vi "Tracker.vi"() -> ()   [LabVIEW 2016]
uses:
  Globaltracker.vi
panel:
  in  "EXPORT 2":enum16{"RAW", "TXT", "CSV"}(ring)
  out "TotalDistanceTraveled":dbl=0.1124215336624257
  out "SegmentsRecalculation":bool[](array[boolean])
  out "ForAnalysisLastRecordingPath":path=path "D:/Users/Dmitriy/CData/CloudStation/Tracker_repository/SavedTrack-2018-02-26-17-00-54/SavedTrack-2018-02-26-17-00-54.csv"
  in  "i":i32=113
  out "NotificationCount":i32
  out "Alarm":dbl caption="minutes" format="%#g"
  out "Loadedregions":picture
  out "Mousebackground":picture
  out "OutsideaSegment":dbl[](array[slide]) scale=-1.0..83.73750000001033
  out "InsideaSegment":dbl[](array[slide]) scale=-1.0..83.73750000001033
  out "TtlArray":T1(array[cluster])
  in  "Main TabControl":enum32{"Settings", "Recording", "Analysis"}(tab)
  in  "CageSegmentation":enum32{"Page 1", "Page 2"}(tab)
  in  "Startup via TTL input 2":bool
  in  "Start/stop signaling":bool=TRUE
  out "CageSegmentation":string="Cage Segmentation"
  out "AssignedSegments":string="Assigned Segments:"
  in  "ListboxOfSegments":i32(listbox)
  in  "Border":enum32{"Page 1", "Page 2"}(tab)
  out "Border":string="BORDER"
  in  "Border":enum16{"8", "6", "5", "4", "3", "2", "1", "0"}(ring)=enum."4" caption="Number of\n segments"
  in  "StartingAngleBorder":u16 caption="Starting\n angle" max=360 step=1
  in  "Center":enum32{"Page 1", "Page 2"}(tab)
  in  "Center":enum16{"1", "0"}(ring) caption="Number of\n segments"
  in  "RadiusCenter":u16=25 caption="Radius \n (mm)" max=90
  out "Center":string="CENTER"
  in  "Midfield":enum32{"Page 1", "Page 2"}(tab)
  in  "StartingAngleMidfield":u32 caption="Starting\n angle" max=360 step=1
  in  "RadiusMidfield":u16=55 caption="Radius\n (mm)" max=90 step=1
  in  "Midfield":enum16{"4", "3", "2", "1", "0"}(ring)=enum."1" caption="Number of\n segments"
  out "Midfiled":string="MIDFIELD"
  out "SettingsDisplay":picture
  out "?":picture
  in  "KeyboardShortcuts":enum32{"Page 1", "Page 2"}(tab)
  out "KeyboardShortcuts":string="Keyboard Shortcuts"
  out "_Assigning Buttons_":bool
  in  "KeyBoardShortCuts":bool
  in  "Notifications":enum32{"Page 1", "Page 2"}(tab)
  out "Notifications":string="Notifications"
  out "Notification":bool
  in  "NotificationsON":bool
  in  "FilterType":enum32{"Page 1", "Page 2"}(tab)
  out "FIlterType":string="Filter Type"
  in  "FilterType":enum16{"No filter", "Kalman filter"}(ring)=enum."Kalman filter"
  in  "PortSelection":enum32{"Page 1", "Page 2"}(tab)
  out "PortSelection":string="Port Selection"
  in  "Data Port Selection":refnum<visa-resource-name>="Tracker"
  in  "SAVE":bool=TRUE
  out "?":picture
  in  "KeyboardShortcuts":enum32{"Page 1", "Page 2"}(tab)
  in  "SegmentsMulticolumnListbox":i32(listbox)
  out "KeyboardShortcuts":string="Keyboard Shortcuts"
  out "Notification":bool
  out "RecordingDisplay":picture
  in  "Cage Segments":enum32{"Page 1", "Page 2"}(tab)
  out "Segments(s)":dbl[](array[slide])=[0.0, 0.0, 0.0, 0.0, 0.0, 4.212500000000026] scale=-1.0..16.81249999999958
  out "Segments":bool[](array[boolean])=[FALSE, FALSE, FALSE, FALSE, FALSE, TRUE]
  out "1":string="1"
  out "2":string="2"
  out "3":string="3"
  out "4":string="4"
  out "5":string="5"
  out "6":string="6"
  out "7":string="7"
  out "8":string="8"
  out "9":string="9"
  out "10\n10":string="10"
  out "11":string="11"
  out "12":string="12"
  out "13":string="13"
  out "CageSegments":string="Cage Segments"
  in  "Cage orientation swap":bool caption="Swap coords"
  in  "RecordingTab":enum32{"Page 1", "Page 2"}(tab)
  out "TTL1 rec armed":bool=TRUE
  in  "Stop Button":bool
  in  "Start":bool
  in  "Trace length (s)":dbl(slide) scale=0.0..10.0
  in  "DisplaySegments":enum32{"Page 1", "Page 2"}(tab)
  in  "DisplaySegments":bool caption="Display Segments"
  out "DisplaySegments":string="Display \nSegments"
  in  "CurrentDistanceTraveled":enum32{"Page 1", "Page 2"}(tab)
  out "Current distance\n traveled (m)":dbl(slide)=0.1124215336624257 scale=0.0..8.0
  out "CurrentDistanceTraveled":string="Current Distance Traveled"
  in  "ElapsedTimeRecording":enum32{"Page 1", "Page 2"}(tab)
  out "Time1":string="           HH:MM:SS,MS"
  out "Time elapsed":string="00:00:04,754"
  out "ElapsedTimeRecording":string="  Elapsed Time (recording)"
  out "Mouse speed (cm/s)":dbl(knob)=3.912345932114511 scale=0.0..100.0 scale format="%#_6f"
  out "Mouse speed (cm/s)  2":dbl(graph)=3.912345932114511 caption="Mouse speed plotted vs time"
  in  "LoadRecording":enum32{"Page 1", "Page 2"}(tab)
  out "FileName":string
  out "ProgressBar":u16(slide) scale=0.0..100.0
  in  "LOAD RECORDING":bool
  in  "ElapsedTimePlayback":enum32{"Page 1", "Page 2"}(tab)
  out "Time2":string="           HH:MM:SS,MS"
  out "ElapsedTimePlayback":string="  Elapsed Time (playback)"
  out "date/time":string
  in  "PlaybackControl":enum32{"Page 1", "Page 2"}(tab)
  in  "Stop Button":bool
  in  "Start/play":bool
  in  "Skip Back Button":bool
  in  "Seek Back Button":bool
  in  "Seek Forward Button":bool
  in  "Skip Forward Button":bool
  in  "Playback progress (min)":dbl(slide) min=0.0 max=24.0 scale=0.0..1.0
  out "Display Speed":dbl
  out "Playback Speed":string="1 X"
  in  "SubtractButton":bool
  in  "AddButton":bool
  out "AnalysisDisplay":picture
  out "Mouse Speed plotted vs time":dbl(graph) caption="Mouse Speed Plotted vs Time"
  out "Mouse speed (cm/s)":dbl(knob) scale=0.0..100.0
  in  "DisplayOptions":enum32{"Page 1", "Page 2"}(tab)
  in  "Heat Map":bool
  in  "Trace_length (s)":dbl(slide) scale=0.0..10.0
  in  "FullTrack":bool caption="Full Track"
  in  "SegmentsOn":bool caption="Segments"
  out "DisplayOptions":string="Display Options"
  in  "Statistics":enum32{"Page 1", "Page 2"}(tab)
  out "Current Distance\n Traveled (m)":dbl(slide) scale=0.0..2.0 scale format="%#_6f"
  out "Total Distance Traveled (m)":dbl
  out "Average Speed (cm/s)":dbl
  out "TTL":bool
  out "Statitics":string="Statistics"
  in  "EXIT":bool=TRUE
  out "index":i32
  out "?":picture
  in  "TimeSpentinEachSegment":enum32{"Page 1", "Page 2"}(tab)
  out "TimeSpentinEachSegment":string="Time Spent in Each Segment"
  in  "TimeSpentinEachSegmentMultiListBox":i32(listbox)=-1
  out "Heat-Map":dbl[][](graph)
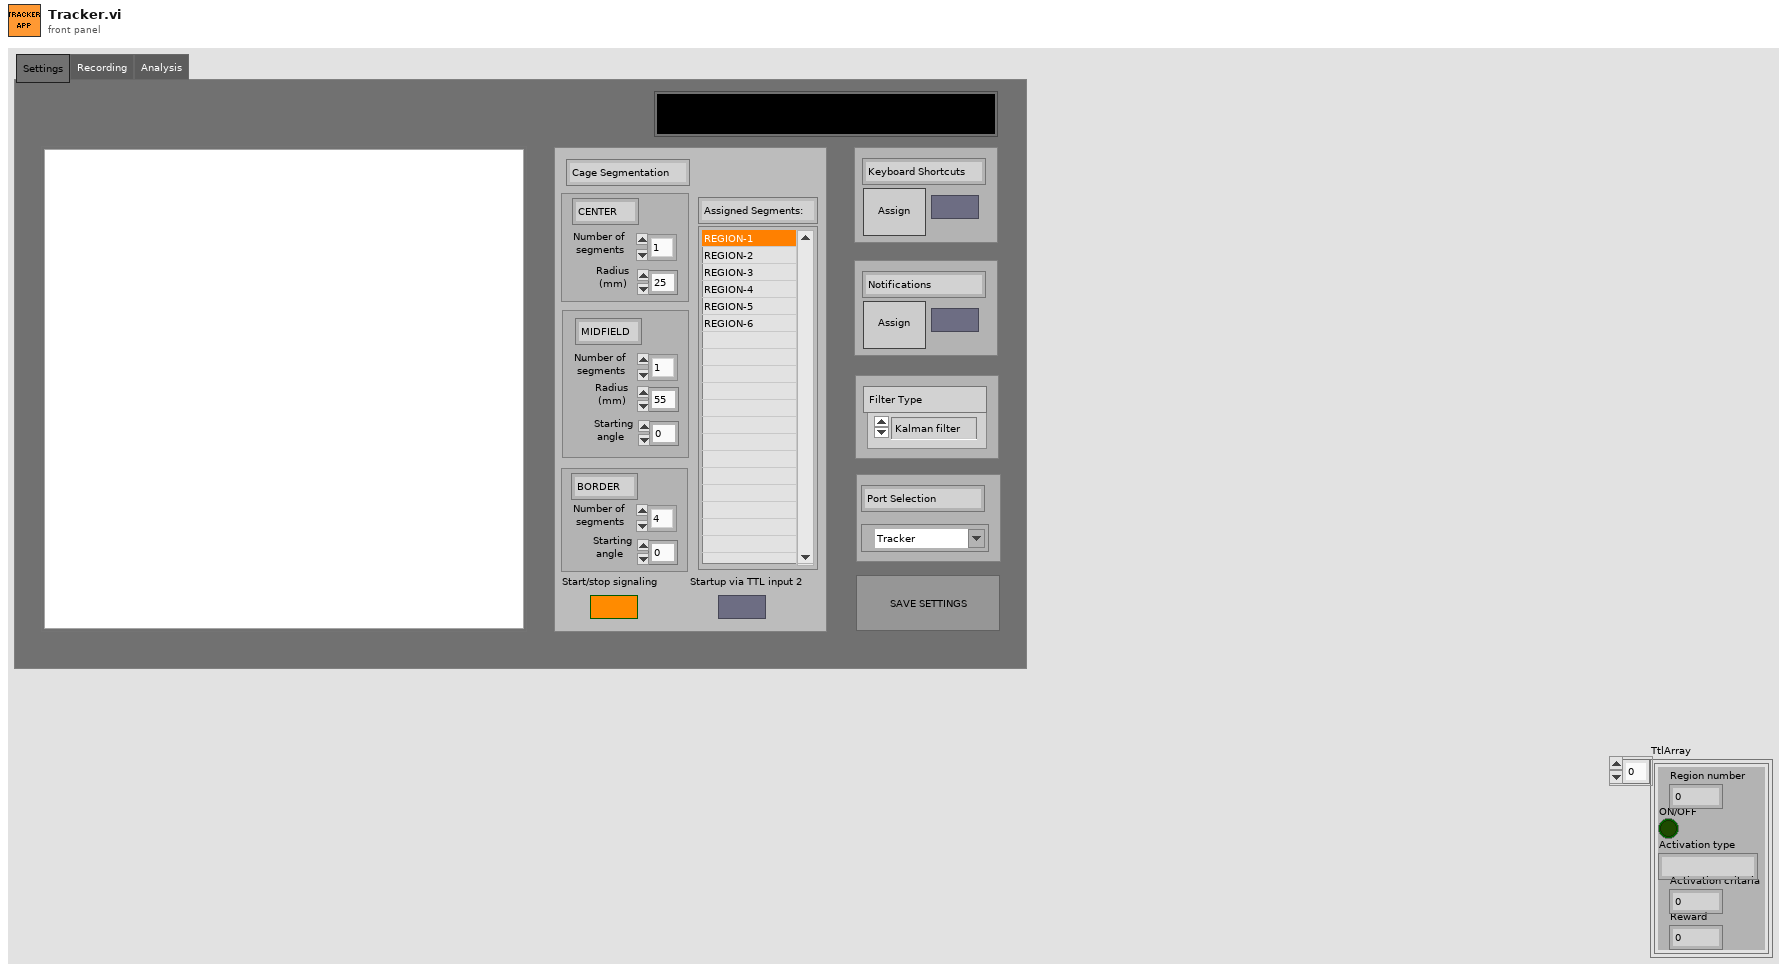
[diagram p1: front panel]
types:
  T1 = cluster{"Region number":i32, "ON/OFF":bool, "Activation type":string, "Activation critaria":i32, "Reward":i32}[]
  T2 = enum16{"No filter", "Kalman filter", "Thresholding"}
  T3 = enum8{"Enabled", "Disabled", "Disabled and Grayed Out"}
  T4 = cluster{"Starting degree of walll":u16, "RewardSystem-ON/OFF":bool, "Image Name":string, "Starting degree of walll":u16, "Starting degree of walll":u16}
  T5 = cluster{"Starting degree of walll":u16, "RewardSystem-ON/OFF":bool, "Image Name":string, "Starting degree of walll":u16, "Starting degree of walll":u16}[]
  T6 = cluster{i32, "ON-OFF":bool, "Activation":string, "ActivationCritaria":i32, "TTLActivation":i32}
  T7 = typedef "imagedata.ctl" = cluster{"image type":i32, "image depth":i32, "image":u8[], "mask":u8[], "colors":u32[], "Rectangle":cluster{"left":i16, "top":i16, "right":i16, "bottom":i16}}
  T8 = typedef "LVMouseTypeDef.ctl" = cluster{"Mouse Position":cluster{"X":i32, "Y":i32}, "Mouse Modifiers":cluster{"Button Down":bool, "Shift Mod":bool, "Menu Mod":bool, "Option Mod":bool}}
  T9 = enum32{"invalid app kind", "Development System", "Run Time System", "Student Edition", "Embedded LabVIEW", "Evaluation", "Custom"}
  T10 = typedef "LVDateTimeRec.ctl" = cluster{"fractional second":dbl, "second":i32, "minute":i32, "hour":i32, "day of month":i32, "month":i32, "year":i32, "day of week":i32, "day of year":i32, "DST":i32}
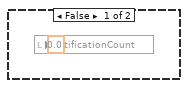
[diagram p2: hidden frame]
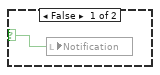
[diagram p4: hidden frame]
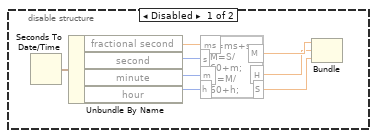
[diagram p6: hidden frame]
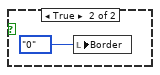
[diagram p9: hidden frame]
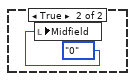
[diagram p10: hidden frame]
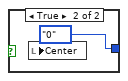
[diagram p11: hidden frame]
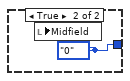
[diagram p12: hidden frame]
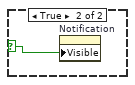
[diagram p14: hidden frame]
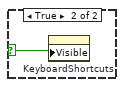
[diagram p15: hidden frame]
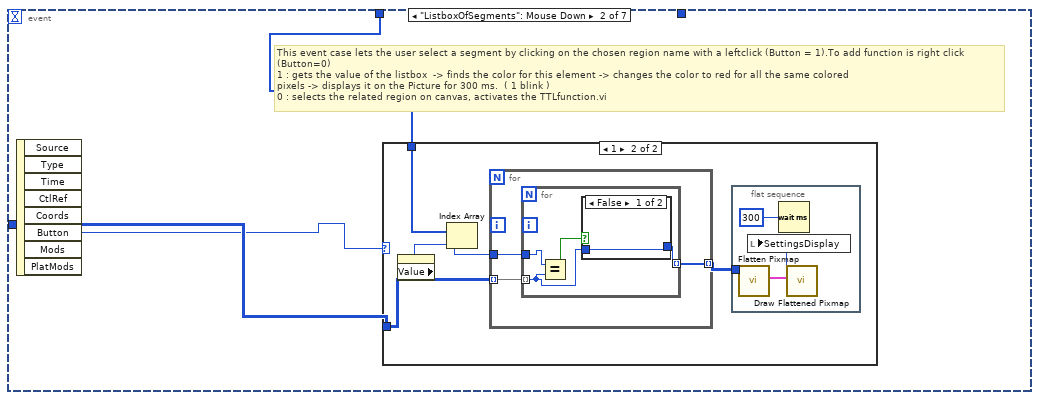
[diagram p16: hidden frame]
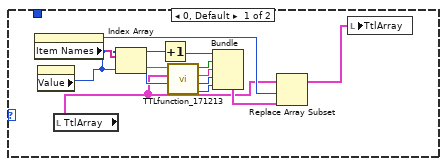
[diagram p17: hidden frame]
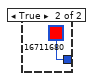
[diagram p18: hidden frame]
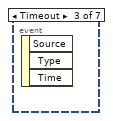
[diagram p19: hidden frame]
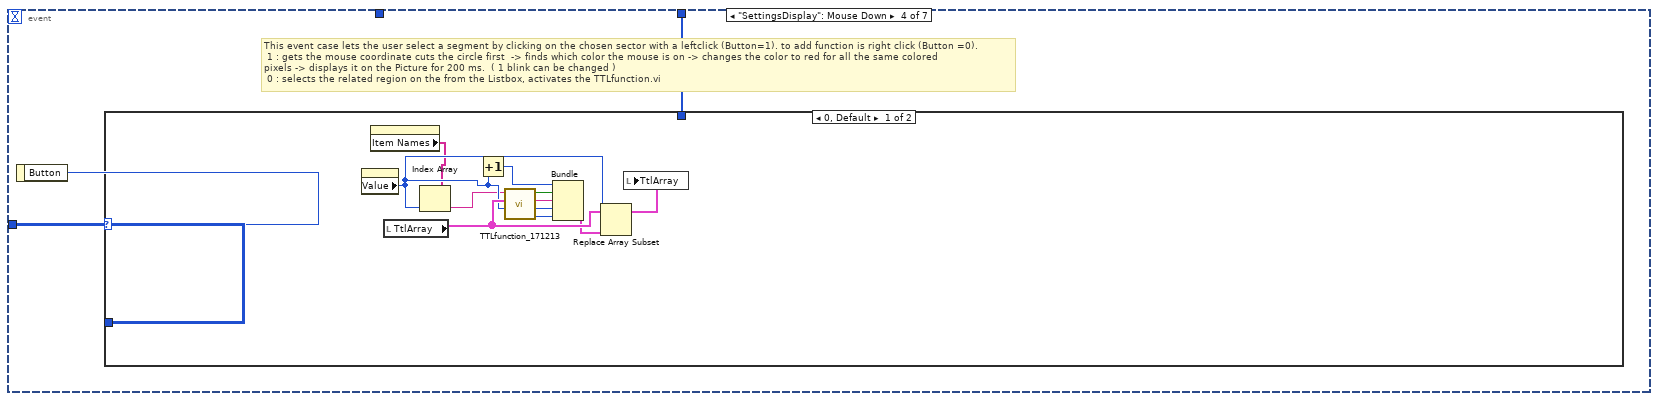
[diagram p20: hidden frame]
diagram:
  # "After-Exit activities"
  n1 = disable-structure shown="Disabled" {
    frame Disabled {
      # "This disabled notification funtion is disabled but can be put back in the \nprogram with and indicator on the screen to make the notifications \navailable in the program. It has a defined \"not moving\" speed and it \ncounts the iteration which are below that speed."
      # "ALARM\nFUNCTION"
      # "speed"
      n2 = Less Or Equal?(y=10.0) -> (x <= y?=w3:bool)  [unwired: 1 in]
      n3 = case shown="True" w3 {
        frame False {
          n4 = local write "NotificationCount"(0.0 ("alarm count")) -> ()
        }
        frame True {
          n5 = local read "NotificationCount"() -> (w8:i32)
          n6 = Increment(x=w8) -> (x+1=w5:i32)
          "NotificationCount" <- w5
          n7 = local read "Alarm"() -> (w7:dbl)
          n8 = Greater Or Equal?(x=w5, y=w7) -> (x >= y?=w6:bool)
          n9 = case shown="True" w6 {
            tunnel: w5 -> [_ w12]
            frame False {
            }
            frame True {
              n10 = To Byte Integer(number=w12) -> (8bit integer=w9:i8)
              n11 = Greater Or Equal?(x=w9, y=i8 0) -> (x >= y?=w11:bool)
              n12 = case shown="True" w11 {
                selector: w11 -> [w13 w14]
                frame False {
                  n13 = local write "Notification"(w13) -> ()
                }
                frame True {
                  "Notification" <- w14
                }
              }
            }
          }
        }
      }
    }
    frame Enabled {
    }
  }
  n14 = flat-sequence {
    tunnel: [w50] -> w1
    tunnel: w1 -> [w55]
    frame #0 {
      w15 = T3."Disabled and Grayed Out" ("Disabled")
      w49 = FALSE ("FULL TRACK")
      # "variables which have\ndefault state"
      # "Static strings : There are so many of them \nFIND option from front panel helps to find the \none\nMany Tabcontrols were used to creat blocks \non the front panel they dont have any fuctions\nexpect the Main TabControl, which is not in the\npile."
      # "These control button are never \nused to read."
      # "THIS FRAME SET THE BASIC DEFAULT STATE FOR THE PROGRAM IT RUNS ONLY ONCE AFTER THE FIRST RUN\nTHEN WE ENTER THE PROGRAM LOOP."
      # "logos"
      n15 = call "StaticStrings2_171213.vi"() -> ("Port Selection"=→"PortSelection":string, "Display"=→"DisplaySegments":string, "2"=→"2":string, "6"=→"6":string, "Midfield"=→"Midfiled":string, "7"=→"7":string, "Notifications"=→"Notifications":string, "1"=→"1":string, "9"=→"9":string)  [unwired: 7 in]
      n16 = global write "Globaltracker.vi" "Analysiss"(w49) -> ()
      n17 = global write "Globaltracker.vi" "NoFilter"(w49) -> ()
      n18 = global write "Globaltracker.vi" "Kalmanfilter"(w49) -> ()
      n19 = local write "SegmentsOn"(w49) -> ()
      n20 = local write "SAVE"(w49) -> ()
      n21 = local write "EXIT"(w49) -> ()
      n22 = global write "Globaltracker.vi" "K"(0.3 ("Threshold")) -> ()
      n23 = local write "Main TabControl"(enum32{"Settings", "Recording", "Analysis"}."Settings" ("Main TabControl")) -> ()
      n24 = property on="Startup via TTL input 2" class="Bool (strict)"("DisabledEnum"=w15) -> ()  [unwired: 2 in, 2 out]
      n25 = property on="Start/stop signaling" class="Bool (strict)"("DisabledEnum"=w15) -> ()  [unwired: 2 in, 2 out]
      n26 = local write "FilterType"(T2."Kalman filter" ("FILTER TYPE")) -> ()
      n27 = property on="Center" class="Enum (strict)"("DisabledEnum"=w15) -> ()  [unwired: 2 in, 2 out]
      n28 = property on="Center" class="Str"("DisabledEnum"=w15) -> ()  [unwired: 2 in, 2 out]
      n29 = call "StaticTextIndicatorstoSaveSpaceonBlockdiogram_171213.vi"() -> ("8"=→"8":string, "KeyboardShortcuts"=→"KeyboardShortcuts":string, "KejyboardShortcuts2"=→"KeyboardShortcuts":string, "Statistics"=→"Statitics":string, "FilterType"=→"FIlterType":string, "CageSegments"=→"CageSegments":string, "TimeSpentinEachSegment"=→"TimeSpentinEachSegment":string, "CageSegmentation"=→"CageSegmentation":string, "AssignedSegments"=→"AssignedSegments":string, "Border"=→"Border":string, "Center"=→"Center":string, "CurrentDistanceTraveled"=→"CurrentDistanceTraveled":string, "DisplayOptions"=→"DisplayOptions":string, "3"=→"3":string, "4"=→"4":string, "ElapsedTimePlayback"=→"ElapsedTimePlayback":string, "12"=→"12":string, "13"=→"13":string, "TIme1"=→"Time1":string, "11"=→"11":string, "Time2"=→"Time2":string, "10"=→"10\n10":string, "ElapsedTimeRecording"=→"ElapsedTimeRecording":string, "5"=→"5":string)  [unwired: 4 in]
      n30 = property on="CageSegmentation" class="Str"("DisabledEnum"=w15) -> ()  [unwired: 2 in, 2 out]
      n31 = property on="RadiusCenter" class="DigNum (strict)"("DisabledEnum"=w15) -> ()  [unwired: 2 in, 2 out]
      n32 = property on="Midfiled" class="Str"("DisabledEnum"=w15) -> ()  [unwired: 2 in, 2 out]
      n33 = property on="StartingAngleBorder" class="DigNum (strict)"("DisabledEnum"=w15) -> ()  [unwired: 2 in, 2 out]
      n34 = property on="Border" class="Str"("DisabledEnum"=w15) -> ()  [unwired: 2 in, 2 out]
      n35 = property on="Border" class="Enum (strict)"("DisabledEnum"=w15) -> ()  [unwired: 2 in, 2 out]
      n36 = property on="Midfield" class="Enum (strict)"("DisabledEnum"=w15) -> ()  [unwired: 2 in, 2 out]
      n37 = property on="StartingAngleMidfield" class="DigNum (strict)"("DisabledEnum"=w15) -> ()  [unwired: 2 in, 2 out]
      n38 = property on="RadiusMidfield" class="DigNum (strict)"("DisabledEnum"=w15) -> ()  [unwired: 2 in, 2 out]
      n39 = property on="ListboxOfSegments" class="LstBox (strict)"("DisabledEnum"=w15) -> ()  [unwired: 2 in, 2 out]
      n40 = property on="AssignedSegments" class="Str"("DisabledEnum"=w15) -> ()  [unwired: 2 in, 2 out]
      n41 = property on="KeyboardShortcuts" class="Str"("DisabledEnum"=w15) -> ()  [unwired: 2 in, 2 out]
      n42 = property on="KeyBoardShortCuts" class="Bool (strict)"("DisabledEnum"=w15) -> ()  [unwired: 2 in, 2 out]
      n43 = property on="_Assigning Buttons_" class="Bool"("DisabledEnum"=w15) -> ()  [unwired: 2 in, 2 out]
      n44 = property on="Notifications" class="Str"("DisabledEnum"=w15) -> ()  [unwired: 2 in, 2 out]
      n45 = property on="Notification" class="Bool"("DisabledEnum"=w15) -> ()  [unwired: 2 in, 2 out]
      n46 = call "LoadinTheStaticPictures_171213.vi"() -> ("background"=w50:picture, "logo"=→"?" →"?" →"?":picture)  [unwired: 10 in]
      n47 = property on="NotificationsON" class="Bool (strict)"("DisabledEnum"=w15) -> ()  [unwired: 2 in, 2 out]
      n48 = property on="FIlterType" class="Str"("DisabledEnum"=w15) -> ()  [unwired: 2 in, 2 out]
      n49 = property on="FilterType" class="Enum (strict)"("DisabledEnum"=w15) -> ()  [unwired: 2 in, 2 out]
      n50 = property on="SAVE" class="Bool (strict)"("DisabledEnum"=w15) -> ()  [unwired: 2 in, 2 out]
    }
    frame #1 {
      n51 = while {
        tunnel: w55 -> [w57]
        stop <- w56 stop-if-true
        # "THIS IS THE ACTUAL PROGRAM LOOP ONLY WAY TO FINISH THIS LOOP IS TO PRESS THE EXIT BUTTON. IT EXITS THE APPLICATION."
        n52 = stacked-sequence {
          tunnel: w57 -> [w61 _ _]
          tunnel: [_ _ w520] -> w56
          frame #0 {
            # "Settings tab of main screen"
            n53 = flat-sequence {
              tunnel: [w76] -> w65
              tunnel: w61 -> [w76]
              tunnel: w65 -> [w88]
              tunnel: [w87] -> w64
              tunnel: [w86] -> w63
              tunnel: [w85] -> w62
              tunnel: [w84] -> w60
              tunnel: w64 -> [w246]
              tunnel: w63 -> [w247]
              tunnel: w62 -> [w251]
              tunnel: w60 -> [w248]
              tunnel: [w247] -> w59
              tunnel: [w246] -> w58
              tunnel: w59 -> [w257]
              tunnel: w58 -> [w256]
              frame #0 {
                w69 = u16 0 ("Starting degree of walll")
                w67 = "" ("Image Name")
                w75 = u16 0 ("Starting degree of walll")
                w83 = FALSE ("RewardSystem-ON/OFF")
                # "Default settings for the segments, the TTL control, Keyboardshortcus"
                n54 = local write "NotificationsON"(w83) -> ()
                n55 = local write "KeyBoardShortCuts"(w83) -> ()
                n56 = global write "Globaltracker.vi" "TTLFuncionEnable"(w83) -> ()
                n57 = local write "Notification"(w83) -> ()
                n58 = local write "Border"(enum16{"8", "6", "5", "4", "3", "2", "1", "0"}."4" ("BORDER")) -> ()
                n59 = local write "Midfield"(enum16{"4", "3", "2", "1", "0"}."1" ("MIDFIELD")) -> ()
                n60 = local write "Center"(enum16{"1", "0"}."1" ("CENTER")) -> ()
                n61 = Build Array(w67, w67) -> (w74:string[])
                n62 = Build Array(w67, w67) -> (w72:string[])
                n63 = Bundle("Starting degree of walll"=w69, "RewardSystem-ON/OFF"=FALSE, "Image Name"=w67, "Starting degree of walll"=w69, "Starting degree of walll"=w69) -> (w70:T4)  [unwired: 1 in]
                n64 = global write "Globaltracker.vi" "Defaultsettings"(TRUE) -> ()
                n65 = Build Array(w74, w72) -> (w73:string[][])
                n66 = Build Array(w70, w70, w70, w70, w70, w70, w70, w70, w70, w70, w70, w70, w70) -> (→"TtlArray":T5)
                n67 = local write "RadiusCenter"(u16 25 ("Radius of the center (mm)")) -> ()
                n68 = local write "Alarm"(w75) -> ()
                n69 = local write "StartingAngleBorder"(w75) -> ()
                n70 = local write "StartingAngleMidfield"(w75) -> ()
                n71 = local write "RadiusMidfield"(u16 55 ("Radius of the middfield (mm)")) -> ()
                n72 = global write "Globaltracker.vi" "KeyboardShortCuts"(w73) -> ()
                n73 = property on="ListboxOfSegments" class="LstBox (strict)"("SelColor"=u32 16744448 ("color(black)")) -> ()  [unwired: 2 in, 2 out]
                "_Assigning Buttons_" <- w83
              }
              frame #1 {
                n74 = while {
                  tunnel: [w121] -> w85
                  tunnel: w88 -> [w120]
                  tunnel: [w115] -> w87
                  tunnel: [w117] -> w86
                  tunnel: [w94] -> w84
                  stop <- w110 stop-if-true
                  w98 = u16 90 ("y")
                  # "The program stays in this loop until the settings got saved or the users chages to the analyzing tab."
                  n75 = global read "Globaltracker.vi" "Analysiss"() -> (w109:bool)
                  n76 = global write "Globaltracker.vi" "Start/stop signalling"("Start/stop signaling") -> ()
                  n77 = local read "Main TabControl"() -> (w106:enum32{"Settings", "Recording", "Analysis"})
                  n78 = Greater Or Equal?(x="RadiusCenter", y=w98) -> (x >= y?=w96:bool)
                  n79 = Or(x="SAVE", y=w109) -> (x .or. y?=w110:bool)
                  n80 = Greater Or Equal?(x="RadiusMidfield", y=w98) -> (x >= y?=w100:bool)
                  n81 = Or(x=w100, y=w96) -> (x .or. y?=w99:bool)
                  n82 = Equal?(x=enum32{"Setting", "Recording", "Analysis"}."Analysis", y=w106) -> (x = y?=w108:bool)
                  n83 = case shown="False" w99 {
                    frame False {
                    }
                    frame True {
                      n84 = local write "Border"(enum16{"8", "6", "5", "4", "3", "2", "1", "0"}."0" ("BORDER")) -> ()
                    }
                  }
                  n85 = call "Border_171213.vi"("StartingAngle"="StartingAngleBorder", "Border"="Border", "InputBackground"=w120) -> ("Colors"=w126:u32[], "OutputPicture"=w129:picture)  [unwired: 7 in]
                  n86 = case shown="True" w108 {
                    frame False {
                    }
                    frame True {
                      n87 = local write "LOAD RECORDING"(FALSE ("LOAD")) -> ()
                      n88 = global write "Globaltracker.vi" "Analysiss"(TRUE ("Anal")) -> ()
                    }
                  }
                  n89 = case shown="False" "NotificationsON" {
                    selector: "NotificationsON" -> [w143 w145]
                    frame False {
                      n90 = property on="Notification" class="Bool (strict)"("Visible"=w143) -> ()  [unwired: 2 in, 2 out]
                      n91 = local write "Alarm"(0.0 ("Alarm")) -> ()
                    }
                    frame True {
                      n92 = property on="Notification" class="Bool (strict)"("Visible"=w145) -> ()  [unwired: 2 in, 2 out]
                    }
                  }
                  n93 = global write "Globaltracker.vi" "Startup via TTL input 2"("Startup via TTL input 2") -> ()
                  n94 = Multiply(x="RadiusMidfield", y=u8 2) -> (x*y=w117:u16)
                  n95 = Greater Or Equal?(x="RadiusCenter", y="RadiusMidfield") -> (x >= y?=w102:bool)
                  n96 = Less Or Equal To 0?(x="RadiusMidfield") -> (x <= 0?=w104:bool)
                  n97 = case shown="False" w104 {
                    tunnel: ["Midfield" w140] -> w105
                    frame False {
                    }
                    frame True {
                      w140 = enum16{"4", "3", "2", "1", "0"}."0" ("MIDFIELD")
                      n98 = local write "Midfield"(w140) -> ()
                    }
                  }
                  n99 = call "Middfield_171213.vi"("StartingAngle"="StartingAngleMidfield", "DiameterOfTheMidfield"=w117, "Midfield"=w105, "InputBackground"=w129) -> ("Colors"=w125:u32[], "OutputBackground"=w128:picture)  [unwired: 6 in]
                  n100 = case shown="False" w102 {
                    frame False {
                    }
                    frame True {
                      n101 = local write "Midfield"(enum16{"4", "3", "2", "1", "0"}."0" ("MIDFIELD")) -> ()
                    }
                  }
                  n102 = case shown="False" "KeyBoardShortCuts" {
                    selector: "KeyBoardShortCuts" -> [w147 w151]
                    frame False {
                      w150 = "" ("Image Name")
                      n103 = property on="KeyboardShortcuts" class="TabCtl (strict)"("Visible"=w147) -> ()  [unwired: 2 in, 2 out]
                      n104 = Build Array(w150, w150) -> (w149:string[])
                      n105 = Build Array(w150, w150) -> (w148:string[])
                      n106 = Build Array(w149, w148) -> (w146:string[][])
                      n107 = global write "Globaltracker.vi" "KeyboardShortCuts"(w146) -> ()
                    }
                    frame True {
                      n108 = property on="KeyboardShortcuts" class="TabCtl (strict)"("Visible"=w151) -> ()  [unwired: 2 in, 2 out]
                    }
                  }
                  n109 = Multiply(x="RadiusCenter", y=u8 2) -> (x*y=w115:u16)
                  n110 = Less Or Equal To 0?(x="RadiusCenter") -> (x <= 0?=w103:bool)
                  n111 = global read "Globaltracker.vi" "Defaultsettings"() -> (w93:bool)
                  n112 = case shown="False" w103 {
                    tunnel: ["Center" w138] -> w127
                    frame False {
                    }
                    frame True {
                      w138 = enum16{"1", "0"}."0" ("CENTER")
                      n113 = local write "Center"(w138) -> ()
                    }
                  }
                  n114 = call "Center_171213.vi"("DiameterOfTheCenter"=w115, "Center"=w127, "InputBackground"=w128) -> ("Colors"=w124:u32[], "OutputBackground"=w123:picture)  [unwired: 7 in]
                  n115 = call "SegmentsFinalize_171213.vi"("BorderColor"=w126, "MidfieldColor"=w125, "CenterColor"=w124, "InputBackground"=w123) -> ("TotalNumberOfSegments"=w121:i32, "RegionNameList"=w122:string[], "Outputbackground"=w92:picture, "OutputPixmapforEvents"=w94:u32[][], "ColorArrayforEvents"=w118:u32[])  [unwired: 3 in]
                  n116 = event shown="[0] \"Data Port Selection\": Value Change" {
                    selector: _ -> [_ _ _ _ _ _ _]
                    dyn-events: _ -> [_ _ _ _ _ _ _]
                    timeout: 0 -> [_ _ _ _ _ _ _]
                    tunnel: w94 -> [_ w156 _ w188 _ _ _]
                    tunnel: w118 -> [_ _ _ w187 _ _ _]
                    tunnel: w118 -> [_ w155 _ _ _ _ _]
                    event "Data Port Selection": Value Change {
                      w152 = T3."Enabled" ("Disabled")
                      n117 = event-data() -> ()  [unwired: 1 in, 6 out]
                      n118 = global write "Globaltracker.vi" "Defaultsettings"(FALSE) -> ()
                      n119 = property on="CageSegmentation" class="Str"("DisabledEnum"=w152) -> ()  [unwired: 2 in, 2 out]
                      n120 = property on="Center" class="Str"("DisabledEnum"=w152) -> ()  [unwired: 2 in, 2 out]
                      n121 = property on="Center" class="Enum (strict)"("DisabledEnum"=w152) -> ()  [unwired: 2 in, 2 out]
                      n122 = property on="RadiusCenter" class="DigNum (strict)"("DisabledEnum"=w152) -> ()  [unwired: 2 in, 2 out]
                      n123 = property on="Midfiled" class="Str"("DisabledEnum"=w152) -> ()  [unwired: 2 in, 2 out]
                      n124 = property on="Midfield" class="Enum (strict)"("DisabledEnum"=w152) -> ()  [unwired: 2 in, 2 out]
                      n125 = property on="RadiusMidfield" class="DigNum (strict)"("DisabledEnum"=w152) -> ()  [unwired: 2 in, 2 out]
                      n126 = property on="StartingAngleMidfield" class="DigNum (strict)"("DisabledEnum"=w152) -> ()  [unwired: 2 in, 2 out]
                      n127 = property on="Border" class="Str"("DisabledEnum"=w152) -> ()  [unwired: 2 in, 2 out]
                      n128 = property on="Border" class="Enum (strict)"("DisabledEnum"=w152) -> ()  [unwired: 2 in, 2 out]
                      n129 = property on="StartingAngleBorder" class="DigNum (strict)"("DisabledEnum"=w152) -> ()  [unwired: 2 in, 2 out]
                      n130 = property on="AssignedSegments" class="Str"("DisabledEnum"=w152) -> ()  [unwired: 2 in, 2 out]
                      n131 = property on="ListboxOfSegments" class="LstBox (strict)"("DisabledEnum"=w152) -> ()  [unwired: 2 in, 2 out]
                      n132 = property on="KeyboardShortcuts" class="Str"("DisabledEnum"=w152) -> ()  [unwired: 2 in, 2 out]
                      n133 = property on="_Assigning Buttons_" class="Bool"("DisabledEnum"=w152) -> ()  [unwired: 2 in, 2 out]
                      n134 = property on="KeyBoardShortCuts" class="Bool (strict)"("DisabledEnum"=w152) -> ()  [unwired: 2 in, 2 out]
                      n135 = property on="Notifications" class="Str"("DisabledEnum"=w152) -> ()  [unwired: 2 in, 2 out]
                      n136 = property on="Notification" class="Bool"("DisabledEnum"=w152) -> ()  [unwired: 2 in, 2 out]
                      n137 = property on="NotificationsON" class="Bool (strict)"("DisabledEnum"=w152) -> ()  [unwired: 2 in, 2 out]
                      n138 = property on="FIlterType" class="Str"("DisabledEnum"=w152) -> ()  [unwired: 2 in, 2 out]
                      n139 = property on="FilterType" class="Enum (strict)"("DisabledEnum"=w152) -> ()  [unwired: 2 in, 2 out]
                      n140 = property on="SAVE" class="Bool (strict)"("DisabledEnum"=w152) -> ()  [unwired: 2 in, 2 out]
                      n141 = property on="Start/stop signaling" class="Bool (strict)"("DisabledEnum"=w152) -> ()  [unwired: 2 in, 2 out]
                      n142 = property on="Startup via TTL input 2" class="Bool (strict)"("DisabledEnum"=w152) -> ()  [unwired: 2 in, 2 out]
                    }
                    event "ListboxOfSegments": Mouse Down {
                      # "This event case lets the user select a segment by clicking on the chosen region name with a leftclick (Button = 1).To add function is right click \n(Button=0)\n1 : gets the value of the listbox  -> finds the color for this element -> changes the color to red for all the same colored\npixels -> displays it on the Picture for 300 ms.  ( 1 blink ) \n0 : selects the related region on canvas, activates the TTLfunction.vi"
                      n143 = event-data() -> ("Button"=w154:u16)  [unwired: 1 in, 7 out]
                      n144 = case shown="1" w154 {
                        tunnel: w156 -> [_ w169]
                        tunnel: w155 -> [_ w168]
                        frame 0, Default {
                          n145 = property on="ListboxOfSegments" class="LstBox (strict)"() -> ("Item Names"=w167:string[])  [unwired: 2 in, 2 out]
                          n146 = property on="ListboxOfSegments" class="LstBox (strict)"() -> ("Value"=w159:i32)  [unwired: 2 in, 2 out]
                          n147 = local read "TtlArray"() -> (w158:T1)
                          n148 = Index Array(array=w167, index=w159) -> (element=w166:string)
                          n149 = Increment(x=w159) -> (x+1=w160:i32)
                          n150 = call "TTLfunction_171213.vi"("RegionClicked"=w159, "TTLArray"=w158, "INPUT STRING"=w166) -> ("TTLActivation"=w162:i32, "ActivationCritaria"=w163:i32, "Activation"=w164:string, "ON-OFF"=w165:bool)  [unwired: 5 in]
                          n151 = Bundle(w160, "ON-OFF"=w165, "Activation"=w164, "ActivationCritaria"=w163, "TTLActivation"=w162) -> (w161:T6)  [unwired: 1 in]
                          n152 = Replace Array Subset(array=w158, new element=w161, index=w159) -> (w157:T1)
                          n153 = local write "TtlArray"(w157) -> ()
                        }
                        frame 1 {
                          n154 = property on="ListboxOfSegments" class="LstBox (strict)"() -> ("Value"=w172:i32)  [unwired: 2 in, 2 out]
                          n155 = Index Array(array=w168, index=w172) -> (element=w171:u32)
                          n156 = for {
                            tunnel: w169 -> [w179] mode=indexing
                            tunnel: w171 -> [w178]
                            tunnel: [w177] -> w170 mode=indexing
                            n157 = for {
                              tunnel: w179 -> [w181] mode=indexing
                              tunnel: w178 -> [w182]
                              tunnel: [w180] -> w177 mode=indexing
                              n158 = Equal?(x=w182, y=w181) -> (x = y?=w183:bool)
                              n159 = case shown="False" w183 {
                                tunnel: [w184 u32 16711680 ("color(black)")] -> w180
                                tunnel: w181 -> [w184 _]
                                frame False {
                                }
                                frame True {
                                }
                              }
                            }
                          }
                          n160 = flat-sequence {
                            tunnel: w170 -> [w176]
                            frame #0 {
                              n161 = call <vilib>:"Flatten Pixmap.vi"("24-bit pixmap"=w176) -> ("image data"=w175:T7)  [unwired: 10 in]
                              n162 = Wait (ms)(milliseconds to wait=u32 300) -> ()  [unwired: 1 out]
                              n163 = call <vilib>:"Draw Flattened Pixmap.vi"("image data"=w175) -> ("new picture"=w174:picture)  [unwired: 8 in]
                              n164 = local write "SettingsDisplay"(w174) -> ()
                            }
                          }
                        }
                      }
                    }
                    event Timeout {
                      n165 = event-data() -> ()  [unwired: 1 in, 3 out]
                    }
                    event "SettingsDisplay": Mouse Down {
                      # "This event case lets the user select a segment by clicking on the chosen sector with a leftclick (Button=1). to add function is right click (Button =0).\n 1 : gets the mouse coordinate cuts the circle first  -> finds which color the mouse is on -> changes the color to red for all the same colored\npixels -> displays it on the Picture for 200 ms.  ( 1 blink can be changed )\n 0 : selects the related region on the from the Listbox, activates the TTLfunction.vi"
                      n166 = event-data() -> ("Button"=w186:u16)  [unwired: 1 in]
                      n167 = case shown="0, Default" w186 {
                        tunnel: w188 -> [_ w206]
                        tunnel: w187 -> [_ w202]
                        frame 0, Default {
                          n168 = property on="ListboxOfSegments" class="LstBox (strict)"() -> ("Value"=w198:i32)  [unwired: 2 in, 2 out]
                          n169 = property on="ListboxOfSegments" class="LstBox (strict)"() -> ("Item Names"=w190:string[])  [unwired: 2 in, 2 out]
                          n170 = local read "TtlArray"() -> (w199:T1)
                          n171 = Index Array(array=w190, index=w198) -> (element=w191:string)
                          n172 = Increment(x=w198) -> (x+1=w197:i32)
                          n173 = call "TTLfunction_171213.vi"("RegionClicked"=w198, "TTLArray"=w199, "INPUT STRING"=w191) -> ("TTLActivation"=w195:i32, "ActivationCritaria"=w194:i32, "Activation"=w193:string, "ON-OFF"=w192:bool)  [unwired: 5 in]
                          n174 = Bundle(w197, "ON-OFF"=w192, "Activation"=w193, "ActivationCritaria"=w194, "TTLActivation"=w195) -> (w196:T6)  [unwired: 1 in]
                          n175 = Replace Array Subset(array=w199, new element=w196, index=w198) -> (w189:T1)
                          n176 = local write "TtlArray"(w189) -> ()
                        }
                        frame 1 {
                          n177 = property on="SettingsDisplay" class="Pict"() -> ("Mouse"=w204:T8)  [unwired: 2 in, 2 out]
                          n178 = Unbundle(w204) -> ("Mouse Position"=w203:cluster{"X":i32, "Y":i32})  [unwired: 1 out]
                          n179 = Unbundle(w203) -> ("X"=w200:i32, "Y"=w201:i32)
                          n180 = Index Array(array=w206, index (row)=w201, index (col)=w200) -> (element=w205:u32)
                          n181 = for {
                            tunnel: w206 -> [w216] mode=indexing
                            tunnel: [w215] -> w207 mode=indexing
                            tunnel: w205 -> [w214]
                            tunnel: w205 -> [w213]
                            tunnel: w202 -> [w212]
                            n182 = for {
                              tunnel: w216 -> [w221] mode=indexing
                              tunnel: [w220] -> w215 mode=indexing
                              tunnel: w214 -> [w219]
                              tunnel: w213 -> [w218]
                              tunnel: w212 -> [w217]
                              n183 = Equal?(x=w219, y=w221) -> (x = y?=w222:bool)
                              n184 = case shown="True" w222 {
                                tunnel: [w223 u32 16711680 ("color(black)")] -> w220
                                tunnel: w221 -> [w223 _]
                                tunnel: w218 -> [_ w225]
                                tunnel: w217 -> [_ w224]
                                frame False {
                                }
                                frame True {
                                n185 = Search 1D Array(1D array=w224, element=w225) -> (index of element=w226:i32)  [unwired: 1 in]
                                n186 = property on="ListboxOfSegments" class="LstBox (strict)"("Value"=w226) -> ()  [unwired: 2 in, 2 out]
                                }
                              }
                            }
                          }
                          n187 = call <vilib>:"Flatten Pixmap.vi"("24-bit pixmap"=w207) -> ("image data"=w208:T7)  [unwired: 10 in]
                          n188 = flat-sequence {
                            tunnel: w208 -> [w211]
                            frame #0 {
                              n189 = call <vilib>:"Draw Flattened Pixmap.vi"("image data"=w211) -> ("new picture"=w209:picture)  [unwired: 8 in]
                              n190 = local write "SettingsDisplay"(w209) -> ()
                              n191 = Wait (ms)(milliseconds to wait=u32 200) -> ()  [unwired: 1 out]
                            }
                          }
                        }
                      }
                    }
                    event "_Assigning Buttons_": Mouse Down {
                      n192 = event-data() -> ()  [unwired: 1 in, 8 out]
                      n193 = global read "Globaltracker.vi" "KeyboardShortCuts"() -> (w228:string[][])
                      n194 = call "AssigningButtons_171213.vi"("Input"=w228) -> ("Cancel Button 2"=w230:bool, "outputarray"=w229:string[][])  [unwired: 9 in]
                      n195 = global write "Globaltracker.vi" "KeyboardShortCuts"(w229) -> ()
                      n196 = case shown="True" w230 {
                        frame False {
                          n197 = local write "KeyBoardShortCuts"(TRUE ("Assigning Buttons")) -> ()
                        }
                        frame True {
                          n198 = local write "KeyBoardShortCuts"(FALSE ("Assigning Buttons")) -> ()
                        }
                      }
                    }
                    event "FilterType": Value Change {
                      # "This event case deals with the filter type for the display of the data stream. It asks the user with a custom made prompt up\nwindow to set the coefficient for the chosen filter.  This number also can be the coefficient for the quoaternion rotation ?"
                      n199 = event-data() -> ("NewVal"=w233:enum16{"No filter", "Kalman filter"})  [unwired: 1 in, 5 out]
                      n200 = case shown="\"Kalman filter\"" w233 {
                        frame "No filter", Default {
                          n201 = global write "Globaltracker.vi" "NoFilter"(TRUE ("Nofilter")) -> ()
                        }
                        frame "Kalman filter" {
                          n202 = call "Kalmancoefficient_171213.vi"() -> ("K"=w235:dbl)  [unwired: 17 in, 2 out]
                          n203 = global write "Globaltracker.vi" "Kalmanfilter"(TRUE ("Nofilter")) -> ()
                          n204 = global write "Globaltracker.vi" "K"(w235) -> ()
                          n205 = global write "Globaltracker.vi" "NoFilter"(FALSE ("Nofilter")) -> ()
                        }
                      }
                    }
                    event "Notification": Mouse Down {
                      # "Converting from minutes to actual iteration number."
                      # "This event case is for the notifications. NOT IN FULL FUNCTION NOW\n This function has to be further developed with additional options for useres.\nNow it would watch the speed of the mouse if it is under a certain value for a given time period then it actives a \"heads\nups\" indicator on the screen."
                      n206 = event-data() -> ()  [unwired: 1 in, 8 out]
                      n207 = call "Alarm_171213.vi"() -> ("CANCEL"=w238:bool, "minutes"=w243:dbl)  [unwired: 16 in, 2 out]
                      n208 = case shown="False" w238 {
                        frame False {
                          n209 = local write "NotificationsON"(TRUE ("_Alarm")) -> ()
                        }
                        frame True {
                          n210 = local write "NotificationsON"(FALSE ("_Alarm")) -> ()
                        }
                      }
                      n211 = Multiply(x=60.0, y=w243) -> (x*y=w242:dbl)
                      n212 = Multiply(x=80.0, y=w242) -> (x*y=→"Alarm":dbl)
                    }
                  }
                  n213 = property on="ListboxOfSegments" class="LstBox (strict)"("Item Names"=w122) -> ()  [unwired: 2 in, 2 out]
                  n214 = case shown="True" w93 {
                    tunnel: w92 -> [w132 w134]
                    tunnel: [w132 w133] -> w91
                    frame False {
                    }
                    frame True {
                      n215 = call "SelectPortonScreen_171213.vi"("input"=w134) -> ("output"=w133:picture)  [unwired: 10 in]
                    }
                  }
                  "SettingsDisplay" <- w91
                }
              }
              frame #2 {
                n216 = global read "Globaltracker.vi" "Analysiss"() -> (w250:bool)
                n217 = local read "TtlArray"() -> (w249:T1)
                n218 = call "PrepareingForRecording_171213.vi"("OutputPixmapforCalculations"=w248, "TTLArray"=w249, "TotalNumberOfSegments"=w251) -> ("Segments(s)"=→"Segments(s)":dbl[], "Segments"=→"Segments" →"SegmentsRecalculation":bool[])  [unwired: 7 in]
                n219 = case shown="False" w250 {
                  frame False {
                    # "Guids the UI for\n the next page"
                    n220 = local write "Main TabControl"(enum32{"Settings", "Recording", "Analysis"}."Recording" ("Main TabControl")) -> ()
                  }
                  frame True {
                    n221 = local write "LOAD RECORDING"(FALSE ("LOAD")) -> ()
                  }
                }
              }
              frame #3 {
                n222 = local read "Midfield"() -> (w261:enum16{"4", "3", "2", "1", "0"})
                n223 = local read "Center"() -> (w262:enum16{"1", "0"})
                n224 = local read "Border"() -> (w260:enum16{"8", "6", "5", "4", "3", "2", "1", "0"})
                n225 = call "Backgrounds_171213.vi"("CENTER"=w262, "DiameterOfTheMidfield"=w257, "DiaMeterOfTheCenter"=w256, "MIDFIELD"=w261, "BORDER"=w260) -> ("OutputMouseBackground"=→"Mousebackground":picture, "NumberedOutput"=w258:picture)  [unwired: 5 in]
                "Loadedregions" <- w258
                n226 = local write "RecordingDisplay"(w258) -> ()
              }
            }
          }
          frame #1 {
            # "Recording tab of main screen"
            n227 = global read "Globaltracker.vi" "Analysiss"() -> (w263:bool)
            n228 = case shown="False" w263 {
              frame False {
                n229 = call "Tracker_hardware_setup.vi"("VISA resource name"="Data Port Selection", "Close port? (T)"=FALSE ("Close port")) -> ("VISA resource name out"=w268:refnum<visa-resource-name>, "ReadStatus"=w265:refnum<notifier>, "error"=w269:bool, "Record_flag"=w264:refnum<notifier>)  [unwired: 4 in, 1 out]
                n230 = case shown="False" w269 {
                  selector: w269 -> [_ w515]
                  tunnel: w265 -> [w288 _]
                  tunnel: w264 -> [w287 _]
                  tunnel: w268 -> [w286 _]
                  frame False {
                    n231 = global read "Globaltracker.vi" "Startup via TTL input 2"() -> (w270:bool)
                    n232 = property on="TTL1 rec armed" class="Bool (strict)"("Blinking"=w270, "Value"=FALSE ("TTL1 rec armed")) -> ()  [unwired: 2 in, 2 out]
                    n233 = flat-sequence {
                      tunnel: [w310] -> w294
                      tunnel: [w312] -> w293
                      tunnel: w288 -> [w299]
                      tunnel: w287 -> [w310]
                      tunnel: w286 -> [w298]
                      tunnel: [w309] -> w284
                      tunnel: [w308] -> w282
                      tunnel: [i32[] [] ("Y out")] -> w281
                      tunnel: [w305] -> w280
                      tunnel: [w304] -> w279
                      tunnel: [w303] -> w278
                      tunnel: [w302] -> w277
                      tunnel: [w301] -> w276
                      tunnel: [w301] -> w275
                      tunnel: [w300] -> w274
                      tunnel: [w297] -> w272
                      tunnel: [w296] -> w271
                      tunnel: w270 -> [w295]
                      tunnel: w294 -> [w344]
                      tunnel: w293 -> [w350]
                      tunnel: [w352] -> w292
                      tunnel: [w362] -> w291
                      tunnel: [w353] -> w290
                      tunnel: [w346] -> w289
                      tunnel: [w361] -> w285
                      tunnel: w284 -> [w360]
                      tunnel: [w359] -> w283
                      tunnel: w282 -> [w359]
                      tunnel: w281 -> [w358]
                      tunnel: w280 -> [w357]
                      tunnel: w279 -> [w356]
                      tunnel: w278 -> [w355]
                      tunnel: w277 -> [w354]
                      tunnel: w276 -> [w353]
                      tunnel: w275 -> [w351]
                      tunnel: w274 -> [w352]
                      tunnel: w272 -> [w343]
                      tunnel: w271 -> [w342]
                      tunnel: w292 -> [w492]
                      tunnel: w291 -> [_]
                      tunnel: w290 -> [w491]
                      tunnel: w289 -> [w496]
                      tunnel: w285 -> [w493]
                      tunnel: w283 -> [w494]
                      frame #0 {
                        w307 = 0.0 ("SUM PATH ( m)")
                        w313 = FALSE ("VISIBLE REGIONS")
                        # "Set most the used displayes and variable to default"
                        n234 = while {
                          tunnel: [w318] -> w312
                          tunnel: [w325] -> w309
                          tunnel: [w325] -> w308
                          tunnel: w299 -> [w322]
                          tunnel: w298 -> [w321]
                          tunnel: [w320] -> w297
                          tunnel: [w319] -> w296
                          tunnel: w295 -> [w316]
                          stop <- w323 stop-if-true
                          # "Allows the user to go back to\nsettings before pressing \nRECORD"
                          n235 = local read "Main TabControl"() -> (w328:enum32{"Settings", "Recording", "Analysis"})
                          n236 = case shown="True" w316 {
                            tunnel: w322 -> [w330 w337]
                            tunnel: w321 -> [w329 w336]
                            tunnel: [w330 w334] -> w320
                            tunnel: [w329 w333] -> w319
                            tunnel: [FALSE ("Start acquisition") w332] -> w317
                            frame False {
                            }
                            frame True {
                              n237 = call "Get_TTL_pulse_length_at_input_2_and_start.vi"("TTL pulse length to trigger start, ms"=200.0, "ReadStatus in"=w337, "VISA resource name"=w336) -> ("Start acquisition"=w332:bool, "ReadStatus out"=w334:refnum<notifier>, "VISA resource name out"=w333:refnum<visa-resource-name>)  [unwired: 5 in, 1 out]
                            }
                          }
                          n238 = Or(x=w317, y="Start") -> (x .or. y?=w318:bool)
                          n239 = Equal?(x=w328, y=enum32{"Setting", "Recording", "Analysis"}."Setting") -> (x = y?=w325:bool)
                          n240 = Or(x=w318, y=w325) -> (x .or. y?=w324:bool)
                          n241 = global write "Globaltracker.vi" "TrackerDisabled"(w325) -> ()
                          n242 = case shown="True" w324 {
                            tunnel: w324 -> [w338 w339]
                            tunnel: [w338 w339] -> w323
                            frame False {
                            }
                            frame True {
                              n243 = property on="TTL1 rec armed" class="Bool (strict)"("Blinking"=FALSE, "Value"=TRUE ("TTL1 rec armed")) -> ()  [unwired: 2 in, 2 out]
                            }
                          }
                        }
                        n244 = local write "NotificationCount"(w307) -> ()
                        n245 = local write "Mouse speed (cm/s)"(w307) -> ()
                        n246 = local write "i"(w307) -> ()
                        n247 = global write "Globaltracker.vi" "TTLSignalActive"(w313) -> ()
                        n248 = property on="Mouse speed (cm/s)  2" class="WFChart (strict)"("History Data"=dbl[] []) -> ()  [unwired: 2 in, 2 out]
                        n249 = local write "Notification"(w313) -> ()
                        n250 = global write "Globaltracker.vi" "Done"(w313) -> ()
                        n251 = local write "Time elapsed"("00:00:00.000" ("date/time string")) -> ()
                        n252 = local read "Segments(s)"() -> (→"InsideaSegment" →"OutsideaSegment":dbl[])
                        n253 = local read "Mousebackground"() -> (w305:picture)
                        n254 = local read "Loadedregions"() -> (w304:picture)
                        n255 = local read "Segments(s)"() -> (w302:dbl[])
                        n256 = local read "Segments"() -> (w303:bool[])
                        n257 = call "Get_temporary_save_path_171213.vi"() -> ("Temporary file output path"=w301:path, "date/time string"=w300:string)  [unwired: 2 in]
                        "TotalDistanceTraveled" <- w307
                        "Current distance\n traveled (m)" <- w307
                      }
                      frame #1 {
                        # "This VI fires approximately 400 ms TTL High on TTL2 output when \"Stop\" button is presssed."
                        # "This VI fires approximately 250 ms TTL High on TTL2 output when \"Record\" button is presssed."
                        n258 = call "Fire_TTL_at_start_stop.vi"("Serial Port In"=w342, "TTL pulse length, ms"=250.0, "Start/stop in"=w350) -> ("Start/stop out"=w349:bool)  [unwired: 6 in, 2 out]
                        n259 = case shown="False" w360 {
                          tunnel: w344 -> [w379 w490]
                          tunnel: w349 -> [w366 _]
                          tunnel: [w378 w490] -> w362
                          tunnel: [w377 w489] -> w346
                          tunnel: w342 -> [w363 w489]
                          tunnel: [w374 w488] -> w361
                          tunnel: w358 -> [w372 _]
                          tunnel: w357 -> [w371 _]
                          tunnel: w356 -> [w370 _]
                          tunnel: w355 -> [w369 _]
                          tunnel: w354 -> [w368 _]
                          tunnel: w351 -> [w367 _]
                          tunnel: [w365 TRUE] -> w348
                          tunnel: w343 -> [w364 _]
                          frame False {
                            # "This main loop is the actual recording period. It terminates if the STOP button is pressed or the Tracker is not connected or does not send the signals.  There is a saving procedure (Save_incrementally.vi)  in this loop which save every data without any additional calculations. \nFurthermore it checks a random ( i = 88)  signal  is correct or not from the tracker if it is not correct the loop terminates and the program displays an error message. (TrackerDisabled case structure)\nOtherwise the streamed data is going to be represented on the screen. On the screen the program only displays every third iteration in order to\ngain speed to the program and it is still over 26 fps display which seems continiuos for a human eye. (other case structure)"
                            n260 = global read "Globaltracker.vi" "TTLFuncionEnable"() -> (w375:bool)
                            n261 = local read "KeyBoardShortCuts"() -> (w373:bool)
                            n262 = local write "Start/play"(FALSE ("Start/play")) -> ()
                            n263 = case shown="True" w373 {
                              frame False {
                              }
                              frame True {
                                n264 = call "Keyboardshortcuts_171213.vi"() -> ()  [unwired: 12 in]
                              }
                            }
                            n265 = case shown="True" w375 {
                              tunnel: w363 -> [_ w380]
                              frame False {
                              }
                              frame True {
                                n266 = call "TrackerTTLsignal_171213.vi"("Serial Port"=w380) -> ()  [unwired: 11 in]
                              }
                            }
                            n267 = while {
                              shift-right: [w430] -> w374
                              shift-left: w368 -> [w439]
                              shift-right: [w392] -> _
                              shift-left: w369 -> [w393]
                              shift-right: [w438] -> _
                              shift-left: w368 -> [w437]
                              shift-right: [w435] -> _
                              shift-left: w368 -> [w436]
                              shift-right: [w429] -> _
                              shift-left: w372 -> [w400]
                              shift-right: [w427] -> _
                              shift-left: w372 -> [w428]
                              tunnel: w363 -> [w416]
                              tunnel: w379 -> [w424]
                              tunnel: w366 -> [w422]
                              tunnel: [w423] -> w378
                              tunnel: [w421] -> w377
                              tunnel: [w399] -> w365
                              tunnel: w371 -> [w398]
                              tunnel: w370 -> [w397]
                              tunnel: w367 -> [w396]
                              tunnel: w364 -> [w381]
                              i -> [w390]
                              stop <- w399 stop-if-true
                              w395 = u32 12 ("milliseconds to wait")
                              n268 = global read "Globaltracker.vi" "Startup via TTL input 2"() -> (w382:bool)
                              n269 = global read "Globaltracker.vi" "Start_Time"() -> (w387:timestamp)
                              n270 = call "Stream_data.vi"("VISA resource name in"=w416, "ReadStatus in"=w381, "Play / Pause"=w422, "Read TTL status in"=w382) -> ("VISA Refnum out"=w421:refnum<visa-resource-name>, "Read TTL status out"=w384:bool, "Current time"=w386:timestamp, "read buffer"=w385:string)  [unwired: 5 in, 3 out]
                              n271 = Increment(x=w395) -> (x+1=w394:u32)
                              n272 = call "Digital_Timer.vi"("Start_Time"=w387, "Current_Time"=w386) -> ("Timer_Out"=→"Time elapsed":string)
                              n273 = Wait (ms)(milliseconds to wait=w394) -> ()  [unwired: 1 out]
                              n274 = call "Decode_RAW_to_DEC.vi"("Read TTL status"=w384, "read buffer"=w385) -> ("DEC SGL output"=w383:sgl[][])
                              n275 = call "Save_incrementally_ts.vi"("Temporary file output path"=w396, "Play / Pause"=TRUE, "Sensor read input"=w383, "Loop iteration"=w390, "Loop speed in ms"=w395, "Save every N seconds"=u32 5, "Current_Time"=w386, "Start_Time"=w387) -> ()  [unwired: 6 in, 2 out]
                              n276 = case shown="True" w422 {
                                tunnel: w424 -> [w449 w452]
                                tunnel: [w449 w450] -> w423
                                frame False {
                                }
                                frame True {
                                n277 = Send Notification(notification=1, notifier=w452) -> (notifier out=w450:refnum<notifier>)  [unwired: 1 in, 1 out]
                                }
                              }
                              n278 = call "RecordingDisplayCalculations_171213.vi"("i"=w390, "DeCOutput"=w383) -> ("Rel Y"=w388:sgl, "Rel X"=w389:sgl, "Mouse angle"=w407:sgl)  [unwired: 7 in]
                              n279 = Empty String/Path?(string/path=w385) -> (empty?=w411:bool)
                              n280 = global read "Globaltracker.vi" "NoFilter"() -> (w414:bool)
                              n281 = case shown="False" w414 {
                                tunnel: w389 -> [w446 w447]
                                tunnel: w388 -> [w445 w448]
                                tunnel: w390 -> [w444 _]
                                tunnel: [w443 w447] -> w418
                                tunnel: [w442 w448] -> w417
                                frame False {
                                n282 = call "KalmanforRelX,Y,angle_171213.vi"("i"=w444, "RelY"=w445, "RelX"=w446) -> ("nextY"=w442:dbl, "nextX"=w443:dbl)  [unwired: 6 in, 1 out]
                                }
                                frame True {
                                }
                              }
                              n283 = Equal?(x=w390, y=88) -> (x = y?=w412:bool)
                              n284 = local read "TotalDistanceTraveled"() -> (w419:dbl)
                              n285 = And(x=w412, y=w411) -> (x .and. y?=w410:bool)
                              n286 = call "DisplacementCalc_171213.vi"("TotalDistanceTraveledInput"=w419, "i"=w390, "Y"=w417, "X"=w418) -> ("Speed"=w401:dbl, "TotalDistanceTraveledOutput"=w406:dbl)  [unwired: 6 in]
                              n287 = case shown="True" w410 {
                                frame False {
                                }
                                frame True {
                                n288 = One Button Dialog(message="ERROR:Tracker is not connected") -> ()  [unwired: 1 in, 1 out]
                                n289 = global write "Globaltracker.vi" "TrackerDisabled"(TRUE ("helping")) -> ()
                                }
                              }
                              n290 = local write "TotalDistanceTraveled"(w406) -> ()
                              n291 = Increment(x=w406) -> (x+1=w403:dbl)
                              n292 = call "TransformTo360_171213.vi"("nextY"=w417, "nextX"=w418) -> ("X"=w426:i32, "Y"=w425:i32)  [unwired: 8 in]
                              n293 = Round Toward +Infinity(x=w403) -> (ceil(x): smallest int >= x=w404:dbl)
                              n294 = Multiply(x=4.0, y=w404) -> (x*y=w402:dbl)
                              n295 = call "TheCoordinateColor_171213.vi"("InputSegments"=w393, "X"=w426, "Y"=w425, "InputSegments(s)"=w439) -> ("MATCH index"=w431:i32, "Outputsegments"=w392:bool[], "OutputSegmens(s)"=w430:dbl[])  [unwired: 5 in]
                              n296 = property on="Current distance\n traveled (m)" class="Slide (strict)"("Scale.Maximum"=w402) -> ()  [unwired: 2 in, 2 out]
                              n297 = call "TTLsignalactivation_171213.vi"("Outside in"=w436, "InputcurrentSegement"=w392, "Inside in"=w437, "InputpriviousSegment"=w393, "MATCH index"=w431) -> ("Inside out"=w438:dbl[], "Outside out"=w435:dbl[])  [unwired: 5 in]
                              n298 = Quotient & Remainder(x=w390, y=3.0 ("x")) -> (x-y*floor(x/y)=w434:dbl)  [unwired: 1 out]
                              n299 = Equal To 0?(x=w434) -> (x = 0?=w433:bool)
                              n300 = case shown="True" w433 {
                                tunnel: w401 -> [_ w486]
                                tunnel: w392 -> [_ w485]
                                tunnel: w430 -> [_ w483]
                                tunnel: w406 -> [_ w484]
                                tunnel: w398 -> [_ w481]
                                tunnel: w397 -> [_ w480]
                                tunnel: w426 -> [_ w479]
                                tunnel: w425 -> [_ w478]
                                tunnel: w407 -> [_ w458]
                                tunnel: w401 -> [_ w476]
                                tunnel: w400 -> [w454 w475]
                                tunnel: [w454 w474] -> w429
                                tunnel: w428 -> [w453 w473]
                                tunnel: [w453 w472] -> w427
                                frame False {
                                }
                                frame True {
                                n301 = Subtract(x=w458, y=sgl 180.0) -> (x-y=w460:sgl)
                                n302 = Less Or Equal To 0?(x=w458) -> (x <= 0?=w462:bool)
                                n303 = Add(x=w458, y=sgl 180.0) -> (x+y=w457:sgl)
                                n304 = Select(t=w457, s=w462, f=w460) -> (s? t:f=w461:sgl)
                                n305 = local write "Segments"(w485) -> ()
                                n306 = Select(t=w461, s="Cage orientation swap", f=w458) -> (s? t:f=w463:sgl)
                                n307 = Multiply(x="Trace length (s)", y=26.666) -> (x*y=w466:dbl)
                                n308 = global write "Globaltracker.vi" "Cage orientation swapped"("Cage orientation swap") -> ()
                                n309 = Round To Nearest(number=w466) -> (nearest integer value=w464:dbl)
                                n310 = local write "Segments(s)"(w483) -> ()
                                n311 = global read "Globaltracker.vi" "KeyboardShortCuts"() -> (w468:string[][])
                                n312 = call "RecordingDisplay_171213.vi"("TrackLength"=w464, "Segments"="DisplaySegments", "NormalMousebackgraound"=w481, "BackgroundSegments"=w480, "X"=w479, "Y"=w478, "i"="i", "X in"=w475, "Angle"=w463, "Y in"=w473) -> ("X out"=w474:i32[], "Y out"=w472:i32[], "RecordingDisplay"=→"RecordingDisplay":picture)  [unwired: 7 in]
                                n313 = Add Array Elements(numeric array=w483) -> (sum=w482:dbl)
                                n314 = local write "Current distance\n traveled (m)"(w484) -> ()
                                n315 = Increment(x="i") -> (x+1=w471:i32)
                                n316 = property on="Segements" class="Slide (strict)"("Scale.Maximum"=w482) -> ()  [unwired: 2 in, 2 out]
                                n317 = local write "i"(w471) -> ()
                                n318 = property on="SegmentsMulticolumnListbox" class="MCListbox (strict)"("ItemNames"=w468) -> ()  [unwired: 2 in, 2 out]
                                "Mouse speed (cm/s)" <- w486
                                "Mouse speed (cm/s)  2" <- w476
                                }
                              }
                              n319 = global read "Globaltracker.vi" "TrackerDisabled"() -> (w408:bool)
                              n320 = Or(x=w408, y="Stop Button") -> (x .or. y?=w399:bool)
                              n321 = global write "Globaltracker.vi" "Done"(w399) -> ()
                            }
                          }
                          frame True {
                            # "If the user wants to go back to settings before pressing start the program allows it in this way. Not recording means (pressing the Settings tab control ) to go to analysing page with those globals, which  immidietely sends the user back to the setting page \nand reset the parameters."
                            n322 = local read "Segments(s)"() -> (w488:dbl[])
                          }
                        }
                        n323 = call "Fire_TTL_at_start_stop.vi"("Serial Port In"=w346, "TTL pulse length, ms"=400.0, "Start/stop in"=w348) -> ()  [unwired: 6 in, 3 out]
                      }
                      frame #2 {
                        # "There would be an error to write some command to \nthe Tracker if it is not connected so there is a case\nstructure for this purpose."
                        n324 = case shown="False" w494 {
                          tunnel: w493 -> [w502 _]
                          tunnel: w492 -> [w501 _]
                          tunnel: w491 -> [w500 _]
                          frame False {
                            # "This saves the segments in the\nfolder in .bpm format."
                            n325 = local read "SegmentsRecalculation"() -> (w505:bool[])
                            n326 = local read "Mousebackground"() -> (w497:picture)
                            n327 = control-ref of="ProgressBar"() -> (w506:refnum<vi>)
                            n328 = call "LoadRecalcSave.vi"("Segments"=w505, "Time"=w501, "Segments(s)"=w502, "LoadBackPath"=w500, "Slide in"=w506) -> ("ForAnalysisPath"=→"ForAnalysisLastRecordingPath":path, "ForSegmentsBMP"=w507:path)  [unwired: 5 in]
                            n329 = local write "Main TabControl"(enum32{"Settings", "Recording", "Analysis"}."Analysis" ("Main TabControl")) -> ()
                            n330 = call "Savingscreen_171213.vi"("NormalMouseBackgroundInput"=w497) -> ("Output"=w498:picture)  [unwired: 10 in]
                            n331 = invoke on="Loadedregions" class="Pict" method="Export Image"("File Type"=enum32{"BMP", "EPS", "EMF", "PICT"}."BMP", "Target"=enum32{"File", "Clipboard"}."File", "Path"=w507) -> ()  [unwired: 4 in, 7 out]
                            n332 = local write "AnalysisDisplay"(w498) -> ()
                          }
                          frame True {
                            # "If there was no recording, then there should\nnot be a saving procedure."
                          }
                        }
                        n333 = global read "Globaltracker.vi" "TrackerDisabled"() -> (w495:bool)
                        n334 = case shown="True" w495 {
                          selector: w495 -> [_ w514]
                          tunnel: w496 -> [w513 _]
                          frame False {
                            n335 = Concatenate Strings("O0" ("write buffer"), "\r") -> (w510:string)
                            n336 = VISA Write(VISA resource name=w513, write buffer=w510) -> (VISA resource name out=w509:refnum<visa-resource-name>)  [unwired: 1 in, 2 out]
                            n337 = VISA Close(VISA resource name=w509) -> ()  [unwired: 1 in, 1 out]
                          }
                          frame True {
                            n338 = global write "Globaltracker.vi" "Analysiss"(w514) -> ()
                          }
                        }
                      }
                    }
                  }
                  frame True {
                    # "An error window comes on the screen and tells the problem : The tracker is not connected. After the okay button pressed the program goes to the analysing part\nbecause that is the only thing what a user can do without the tracker."
                    n339 = global write "Globaltracker.vi" "Analysiss"(w515) -> ()
                    n340 = flat-sequence {
                      frame #0 {
                        n341 = One Button Dialog(message="ERROR:Tracker is not connected") -> ()  [unwired: 1 in, 1 out]
                      }
                      frame #1 {
                        n342 = local write "Main TabControl"(enum32{"Settings", "Recording", "Analysis"}."Analysis" ("Main TabControl")) -> ()
                      }
                    }
                  }
                }
              }
              frame True {
                # "If analysis was clicked by the user the program skips the recording part"
                n343 = local write "LOAD RECORDING"(FALSE ("LOAD")) -> ()
              }
            }
          }
          frame #2 {
            # "Analysis tab of main screen"
            n344 = global read "Globaltracker.vi" "Analysiss"() -> (w519:bool)
            n345 = case shown="True" w519 {
              frame False {
                n346 = local write "LOAD RECORDING"(TRUE ("LOAD RECORDING")) -> ()
              }
              frame True {
                n347 = local write "LOAD RECORDING"(FALSE ("LOAD")) -> ()
              }
            }
            n348 = while {
              tunnel: ["EXIT"] -> w520
              tunnel: w519 -> [_]
              stop <- w524 stop-if-true
              # "This is the main loop in the analyzis part. This allows to analyze multiple files until the user exits the program or goes back to setting for a new recording,"
              n349 = case shown="True" "LOAD RECORDING" {
                tunnel: [w529 w546] -> w526
                frame False {
                  w527 = FALSE ("Stop Button 2")
                  w528 = 0.0 ("SUM PATH ( m) 2")
                  w535 = "" ("date/time string A")
                  # "In this case while the program waits for the user to load in a recording. It displays Load a Recording on the canvas. Make all the variables back to default.\nAnd let the user go back to the fistt page ( settings) to make a new recording ( after saving the settings )"
                  n350 = local read "Mousebackground"() -> (w534:picture)
                  n351 = local write "FileName"(w535) -> ()
                  n352 = local write "index"(w528) -> ()
                  n353 = local write "date/time"(w535) -> ()
                  n354 = property on="Mouse Speed plotted vs time" class="WFChart (strict)"("History Data"=dbl[] []) -> ()  [unwired: 2 in, 2 out]
                  n355 = call "LoadRecordingscreen_171213.vi"("Input"=w534) -> ("Output"=w533:picture)  [unwired: 10 in]
                  n356 = property on="Playback progress (min)" class="Slide (strict)"("Scale.Minimum"=w528) -> ()  [unwired: 2 in, 2 out]
                  n357 = local write "AnalysisDisplay"(w533) -> ()
                  n358 = local write "Display Speed"(w528) -> ()
                  n359 = local write "Mouse speed (cm/s)"(w528) -> ()
                  n360 = local write "Average Speed (cm/s)"(w528) -> ()
                  n361 = local write "Playback progress (min)"(w528) -> ()
                  n362 = local write "Playback progress (min)"(w528) -> ()
                  n363 = local write "Total Distance Traveled (m)"(w528) -> ()
                  n364 = global write "Globaltracker.vi" "CounterDownforPlaybackSpeed"(w528) -> ()
                  n365 = global write "Globaltracker.vi" "CounterUpforPlaybackSpeed"(w528) -> ()
                  n366 = local write "Current Distance\n Traveled (m)"(w528) -> ()
                  n367 = local write "Mouse Speed plotted vs time"(w528) -> ()
                  n368 = local write "SubtractButton"(w527) -> ()
                  n369 = global write "Globaltracker.vi" "TrackerDisabled"(w527) -> ()
                  n370 = local write "Stop Button"(w527) -> ()
                  n371 = local write "Seek Back Button"(w527) -> ()
                  n372 = local write "Heat Map"(w527) -> ()
                  n373 = local write "SegmentsOn"(w527) -> ()
                  n374 = local write "AddButton"(w527) -> ()
                  n375 = local write "Skip Back Button"(w527) -> ()
                  n376 = local write "Seek Forward Button"(w527) -> ()
                  n377 = local write "Skip Forward Button"(w527) -> ()
                  n378 = local write "FullTrack"(w527) -> ()
                  n379 = local read "Main TabControl"() -> (w532:enum32{"Settings", "Recording", "Analysis"})
                  n380 = Equal?(x=w532, y=enum32{"Setting", "Recording", "Analysis"}."Setting") -> (x = y?=w531:bool)
                  n381 = case shown="True" w531 {
                    selector: w531 -> [_ w538]
                    tunnel: [FALSE w538] -> w529
                    frame False {
                    }
                    frame True {
                      w539 = FALSE ("HTrackerOff")
                      n382 = global write "Globaltracker.vi" "Analysiss"(w539) -> ()
                      n383 = local write "SAVE"(w539) -> ()
                    }
                  }
                }
                frame True {
                  # "If the user select a file the analyzis steps forward\nif it is cancelled or closes then the analyzing part\nis skipped and the program goes to the waiting\nstate where the new decision can be made by \nthe user. Load another one, exit , or go to setting\nand record a new one."
                  # "This starts also with a case structure because\nidially the program immedietaly loads back \nthe last recording. If it is not the last recording \nthen it waits for the user to select a file."
                  # "This case structure allows to reload or wait for an another decision like exit or new recording or load an other recording"
                  n384 = global read "Globaltracker.vi" "Analysiss"() -> (w544:bool)
                  n385 = Not(x=w544) -> (.not. x?=w545:bool)
                  n386 = case shown="True" w545 {
                    tunnel: [w551 w553] -> w541
                    tunnel: [w547 FALSE ("cancelled")] -> w543
                    frame False {
                      n387 = call "File Dialog"() -> ("selected path"=w551:path, "cancelled"=w548:bool, "error out"=w550:errorcluster)  [unwired: 12 in, 1 out]
                      n388 = Unbundle(w550) -> ("status"=w549:bool)  [unwired: 2 out]
                      n389 = Or(x=w549, y=w548) -> (x .or. y?=w547:bool)
                    }
                    frame True {
                      n390 = local read "ForAnalysisLastRecordingPath"() -> (w553:path)
                    }
                  }
                  n391 = Not(x=w543) -> (.not. x?=w542:bool)
                  n392 = local write "LOAD RECORDING"(w542) -> ()
                  n393 = case shown="True" w542 {
                    tunnel: [FALSE w573] -> w546
                    tunnel: w543 -> [_ w569]
                    tunnel: w541 -> [_ w571]
                    frame False {
                      # "The program goes back to the waiting state:  where the new decision can be made by \nthe user. Load another one, exit , or go to setting and record a new one."
                    }
                    frame True {
                      w555 = FALSE ("Stop Button 2")
                      w558 = 0.0 ("SUM PATH ( m) 2")
                      # "This case structure is the analyzing part before entering a loop the actual playback. It starts with calculation outside of the loop to let the loop run on max iteration speed. And sets the values back to default."
                      n394 = call "ReloadCSVforanalysispart_171213.vi"("Path"=w571) -> ("Clean data array"=w568:dbl[][], "Time"=w572:string[])  [unwired: 1 in, 3 out]
                      n395 = call "LoadFileName_171213.vi"("SelectedPath"=w571) -> ("FIleName"=→"FileName":string)  [unwired: 10 in]
                      n396 = local read "Mousebackground"() -> (w556:picture)
                      n397 = call "Transformationto360x360matrixcoordinates_171213.vi"("FilteredInputData"=w568) -> ("360Y"=w564:dbl[], "360X"=w565:dbl[])  [unwired: 9 in]
                      n398 = property on="Playback progress (min)" class="Slide (strict)"("Scale.Minimum"=w558) -> ()  [unwired: 2 in, 2 out]
                      n399 = local write "Start/play"(w555) -> ()
                      n400 = local write "LOAD RECORDING"(w555) -> ()
                      n401 = local write "Stop Button"(w555) -> ()
                      n402 = local write "Skip Forward Button"(w555) -> ()
                      n403 = local write "Seek Back Button"(w555) -> ()
                      n404 = local write "Heat Map"(w555) -> ()
                      n405 = local write "Skip Back Button"(w555) -> ()
                      n406 = local write "Seek Forward Button"(w555) -> ()
                      n407 = local write "AddButton"(w555) -> ()
                      n408 = local write "FullTrack"(w555) -> ()
                      n409 = local write "FullTrack"(w555) -> ()
                      n410 = local write "SubtractButton"(w555) -> ()
                      n411 = local write "SegmentsOn"(w555) -> ()
                      n412 = global write "Globaltracker.vi" "CounterDownforPlaybackSpeed"(w558) -> ()
                      n413 = global write "Globaltracker.vi" "CounterUpforPlaybackSpeed"(w558) -> ()
                      n414 = local write "Playback progress (min)"(w558) -> ()
                      n415 = property on="Current Distance Traveled (m)" class="Slide (strict)"("Scale.Minimum"=w558) -> ()  [unwired: 2 in, 2 out]
                      n416 = case shown="False" w569 {
                        tunnel: w556 -> [w575 w577]
                        tunnel: [w574 w576] -> w570
                        frame False {
                          n417 = call "Loadingscreen_171213.vi"("2D Picture"=w575) -> ("2D Picture 2"=w574:picture)  [unwired: 10 in]
                        }
                        frame True {
                          n418 = call "LoadRecordingscreen_171213.vi"("Input"=w577) -> ("Output"=w576:picture)  [unwired: 10 in]
                        }
                      }
                      n419 = control-ref of="ProgressBar"() -> (w567:refnum<vi>)
                      n420 = local write "Playback Speed"("1 X" ("Display Speed")) -> ()
                      n421 = call "BackgroundFulltrackCalculations_171213.vi"("360Y"=w564, "Mousebackground"=w556, "360X"=w565, "ForAnalysisLastRecordingPath"=w571, "Slide in"=w567) -> ("BackgroundSegmentforAnalysis"=w566:picture, "NormalMousebackgroundOutput"=w562:picture, "BackgroundSegmentsOutput"=w563:picture, "HeatMap"=→"Heat-Map":dbl[][])  [unwired: 3 in]
                      n422 = local write "AnalysisDisplay"(w570) -> ()
                      n423 = while {
                        tunnel: [FALSE] -> w573
                        tunnel: w568 -> [w594]
                        tunnel: w572 -> [w593]
                        tunnel: w566 -> [w592]
                        tunnel: w564 -> [w591]
                        tunnel: w565 -> [w590]
                        tunnel: w563 -> [w589]
                        tunnel: w562 -> [w588]
                        tunnel: w556 -> [w584]
                        stop <- w587 stop-if-true
                        # "This loop is the analyzing the same file over and over again until the user does not say new file or exists the program or goes back for and other recording."
                        n424 = flat-sequence {
                          tunnel: [w622] -> w602
                          tunnel: [w621] -> w600
                          tunnel: [w620] -> w601
                          tunnel: [w619] -> w599
                          tunnel: [w618] -> w598
                          tunnel: [w617] -> w597
                          tunnel: [w604] -> w596
                          tunnel: w593 -> [w622]
                          tunnel: w592 -> [w621]
                          tunnel: w591 -> [w620]
                          tunnel: w590 -> [w604]
                          tunnel: w594 -> [w607]
                          tunnel: w584 -> [w619]
                          tunnel: w588 -> [w618]
                          tunnel: w589 -> [w617]
                          tunnel: [w615] -> w583
                          tunnel: [w610] -> w582
                          tunnel: [w609] -> w581
                          tunnel: [w608] -> w580
                          tunnel: [i32[] [] ("Y out 5")] -> w579
                          tunnel: [w603] -> w578
                          tunnel: w602 -> [w641]
                          tunnel: w601 -> [w640]
                          tunnel: w600 -> [w639]
                          tunnel: w599 -> [w638]
                          tunnel: w598 -> [w636]
                          tunnel: w597 -> [w637]
                          tunnel: w596 -> [w635]
                          tunnel: [w634] -> w585
                          tunnel: w583 -> [w633]
                          tunnel: w582 -> [w632]
                          tunnel: w581 -> [w631]
                          tunnel: w580 -> [w630]
                          tunnel: w579 -> [w629]
                          tunnel: w578 -> [w628]
                          tunnel: [w804] -> w586
                          tunnel: w585 -> [w804]
                          tunnel: [w809] -> w587
                          tunnel: w586 -> [w808]
                          frame #0 {
                            # "This frame waits for the user to \npress the start button.\nIt displays the constant vaules or sets\nback to default."
                            n425 = call "SumTimeSpendAnalyze_171213.vi"("Clean data array"=w607) -> ("Item Names"=w616:string[][])  [unwired: 10 in]
                            n426 = while {
                              stop <- w625 stop-if-true
                              n427 = local read "Mousebackground"() -> (w627:picture)
                              n428 = local read "EXIT"() -> (w623:bool)
                              n429 = Or(x="Start/play", y=w623) -> (x .or. y?=w625:bool)
                              n430 = call "PressPlay_171213.vi"("Input"=w627) -> ("Output"=w626:picture)  [unwired: 10 in]
                              n431 = local write "AnalysisDisplay"(w626) -> ()
                            }
                            n432 = property on="TimeSpentinEachSegmentMultiListBox" class="MCListbox (strict)"("ItemNames"=w616) -> ()  [unwired: 2 in, 2 out]
                            n433 = property on="Mouse Speed plotted vs time" class="WFChart (strict)"("History Data"=dbl[] []) -> ()  [unwired: 2 in, 2 out]
                            n434 = call "SelectColumnstoPlaybackDisplay_171213.vi"("Clean data array in"=w607) -> ("Speed"=w615:dbl[], "TotalDIstanceTraveled"=w614:dbl, "Playbackprogress(min)maxscale"=w613:dbl, "CurrentDIstancemaxScale"=w612:dbl, "AVGSpeed"=w611:dbl, "CurrentDistanceTraveled"=w610:dbl[], "TTL"=w609:dbl[], "Angle"=w608:dbl[])  [unwired: 3 in]
                            n435 = property on="Playback progress (min)" class="Slide (strict)"("Scale.Maximum"=w613) -> ()  [unwired: 2 in, 2 out]
                            n436 = local write "Total Distance Traveled (m)"(w614) -> ()
                            n437 = local write "Average Speed (cm/s)"(w611) -> ()
                            n438 = property on="Current Distance\n Traveled (m)" class="Slide (strict)"("Scale.Maximum"=w612) -> ()  [unwired: 2 in, 2 out]
                            n439 = Array Size(array=w604) -> (size(s)=w603:i32)
                          }
                          frame #1 {
                            n440 = while {
                              tunnel: w639 -> [w679]
                              shift-right: [w678] -> _
                              shift-left: w629 -> [w677]
                              shift-right: [w676] -> _
                              shift-left: w629 -> [w675]
                              tunnel: w628 -> [w643]
                              tunnel: w641 -> [w651]
                              tunnel: w640 -> [w666]
                              tunnel: w635 -> [w665]
                              tunnel: w638 -> [w650]
                              tunnel: w637 -> [w645]
                              tunnel: w636 -> [w647]
                              tunnel: [w658] -> w634
                              tunnel: w633 -> [w657]
                              tunnel: w632 -> [w656]
                              tunnel: w631 -> [w654]
                              tunnel: w630 -> [w655]
                              stop <- w659 stop-if-true
                              # "This loop is responsible for the analyzing display"
                              n441 = flat-sequence {
                                tunnel: [w698] -> w674
                                tunnel: [w697] -> w673
                                tunnel: [w696] -> w672
                                tunnel: [w689] -> w671
                                tunnel: [w687] -> w670
                                tunnel: [w691] -> w669
                                tunnel: [w692] -> w668
                                tunnel: w679 -> [w698]
                                tunnel: w677 -> [w697]
                                tunnel: w675 -> [w696]
                                tunnel: [w688] -> w667
                                tunnel: w666 -> [w692]
                                tunnel: w665 -> [w691]
                                tunnel: w657 -> [w689]
                                tunnel: w656 -> [w688]
                                tunnel: w655 -> [w687]
                                tunnel: w654 -> [w686]
                                tunnel: [w686] -> w653
                                tunnel: [w685] -> w652
                                tunnel: w651 -> [w685]
                                tunnel: w650 -> [w684]
                                tunnel: [w684] -> w649
                                tunnel: [w683] -> w648
                                tunnel: w647 -> [w683]
                                tunnel: [w682] -> w646
                                tunnel: w645 -> [w682]
                                tunnel: [w681] -> w644
                                tunnel: w643 -> [w681]
                                tunnel: [w729] -> w658
                                tunnel: w674 -> [w763]
                                tunnel: w673 -> [w762]
                                tunnel: w672 -> [w761]
                                tunnel: w671 -> [w759]
                                tunnel: w670 -> [w758]
                                tunnel: w669 -> [w756]
                                tunnel: w668 -> [w754]
                                tunnel: w667 -> [w752]
                                tunnel: [w741] -> w664
                                tunnel: [w739] -> w662
                                tunnel: w653 -> [w716]
                                tunnel: w652 -> [w715]
                                tunnel: w649 -> [w714]
                                tunnel: w648 -> [w713]
                                tunnel: w646 -> [w712]
                                tunnel: w644 -> [w711]
                                tunnel: [w701] -> w642
                                tunnel: w664 -> [w795]
                                tunnel: [w795] -> w663
                                tunnel: w662 -> [w794]
                                tunnel: [w794] -> w661
                                tunnel: w642 -> [w792]
                                tunnel: [w801] -> w678
                                tunnel: [w802] -> w676
                                tunnel: w663 -> [w801]
                                tunnel: w661 -> [w802]
                                frame #0 {
                                n442 = Multiply(x="Playback progress (min)", y=60.0) -> (x*y=w693:dbl)
                                n443 = Multiply(x=w693, y=80) -> (x*y=w680:dbl)
                                n444 = global write "Globaltracker.vi" "index"(w680) -> ()
                                }
                                frame #1 {
                                n445 = case shown="False" "Heat Map" {
                                frame False {
                                n446 = flat-sequence {
                                frame #0 {
                                n447 = property on="AnalysisDisplay" class="Pict"("Visible"=TRUE) -> ()  [unwired: 2 in, 2 out]
                                }
                                frame #1 {
                                n448 = property on="Heat-Map" class="IntGraph (strict)"("Visible"=FALSE) -> ()  [unwired: 2 in, 2 out]
                                }
                                }
                                }
                                frame True {
                                n449 = flat-sequence {
                                frame #0 {
                                n450 = property on="Heat-Map" class="IntGraph (strict)"("Visible"=TRUE) -> ()  [unwired: 2 in, 2 out]
                                }
                                frame #1 {
                                n451 = property on="AnalysisDisplay" class="Pict"("Visible"=FALSE) -> ()  [unwired: 2 in, 2 out]
                                }
                                }
                                }
                                }
                                n452 = global read "Globaltracker.vi" "index"() -> (w703:i32)
                                n453 = Index Array(array=w752, index=w703) -> (element=w751:dbl)
                                n454 = Index Array(array=w759, index=w703) -> (element=w735:dbl)
                                n455 = Index Array(array=w715, index=w703) -> (element=w734:string)
                                n456 = Index Array(array=w716, index=w703) -> (element=w732:dbl)
                                n457 = Index Array(array=w758, index=w703) -> (element=w757:dbl)
                                n458 = Index Array(array=w756, index=w703) -> (element=w755:dbl)
                                n459 = Index Array(array=w754, index=w703) -> (element=w753:dbl)
                                n460 = local write "Current Distance\n Traveled (m)"(w751) -> ()
                                n461 = local write "Mouse speed (cm/s)"(w735) -> ()
                                n462 = local write "date/time"(w734) -> ()
                                n463 = Equal?(x=1.0, y=w732) -> (x = y?=→"TTL":bool)
                                n464 = local write "Mouse Speed plotted vs time"(w735) -> ()
                                n465 = Multiply(x="Trace_length (s)", y=80.0) -> (x*y=w765:dbl)
                                n466 = Round To Nearest(number=w765) -> (nearest integer value=w760:dbl)
                                n467 = Or(x="Skip Forward Button", y="Skip Back Button") -> (x .or. y?=w738:bool)
                                n468 = Or(x="Seek Forward Button", y="Seek Back Button") -> (x .or. y?=w737:bool)
                                n469 = Or(x=w738, y=w737) -> (x .or. y?=w736:bool)
                                n470 = Add(x=w703, y=400) -> (x+y=w749:i32)
                                n471 = Greater Or Equal?(x=w703, y=w711) -> (x >= y?=w733:bool)
                                n472 = control-ref of="Skip Back Button"() -> (w707:refnum<vi>)
                                n473 = case shown="True" w736 {
                                tunnel: w703 -> [_ w775]
                                tunnel: w749 -> [_ w774]
                                frame False {
                                # "This Case straucture is only for the Mouse Speed \nplotted vs Time display. Especially the scale and \nmemory of that indicator. \nIf the users changes time position of the playback\nby using the playback buttons, then the memory of\nthis display indicator is cleared."
                                }
                                frame True {
                                n474 = flat-sequence {
                                tunnel: w775 -> [w778]
                                tunnel: w774 -> [w777]
                                frame #0 {
                                n475 = property on="Mouse Speed plotted vs time" class="WFChart (strict)"("History Data"=dbl[] []) -> ()  [unwired: 2 in, 2 out]
                                }
                                frame #1 {
                                n476 = property on="Mouse Speed plotted vs time" class="WFChart (strict)"("XScale.Maximum"=w777, "XScale.Minimum"=w778) -> ()  [unwired: 2 in, 2 out]
                                }
                                }
                                }
                                }
                                n477 = event shown="[1] \"AddButton\": Mouse Down" {
                                selector: _ -> [_ _ _]
                                dyn-events: _ -> [_ _ _]
                                timeout: 0 -> [_ _ _]
                                event Timeout {
                                n478 = event-data() -> ()  [unwired: 1 in, 3 out]
                                }
                                event "AddButton": Mouse Down {
                                n479 = event-data() -> ()  [unwired: 1 in, 1 out]
                                n480 = global read "Globaltracker.vi" "CounterUpforPlaybackSpeed"() -> (w766:i16)
                                n481 = Increment(x=w766) -> (x+1=w767:i16)
                                n482 = global write "Globaltracker.vi" "CounterUpforPlaybackSpeed"(w767) -> ()
                                }
                                event "SubtractButton": Mouse Down {
                                n483 = event-data() -> ()  [unwired: 1 in, 1 out]
                                n484 = global read "Globaltracker.vi" "CounterDownforPlaybackSpeed"() -> (w768:i16)
                                n485 = Increment(x=w768) -> (x+1=w769:i16)
                                n486 = global write "Globaltracker.vi" "CounterDownforPlaybackSpeed"(w769) -> ()
                                }
                                }
                                n487 = control-ref of="Skip Forward Button"() -> (w706:refnum<vi>)
                                n488 = Or(x="Stop Button", y=w733) -> (x .or. y?=w729:bool)
                                n489 = control-ref of="Seek Back Button"() -> (w705:refnum<vi>)
                                n490 = call "Displayspeed.vi"() -> ("Increment"=w699:dbl, "DisplaySpeed"=w701:dbl, "Waitin(ms)"=w702:dbl)  [unwired: 9 in]
                                n491 = local read "Start/play"() -> (w727:bool)
                                n492 = To Unsigned Word Integer(number=w699) -> (unsigned 16bit integer=w700:u16)
                                n493 = Add(x=w700, y=w703) -> (x+y=w710:i32)
                                n494 = call "AnalysisDisplay_171213.vi"("TraceLength"=w760, "Segments"="SegmentsOn", "FullTrack"="FullTrack", "FulltrackonBackgroundSegments"=w712, "BackgroundSegments"=w763, "NormalMouseBackground"=w714, "X"=w755, "Y"=w753, "i"=w710, "X in"=w762, "Angle"=w757, "Y in"=w761, "FulltrackonNormalMouseBackground"=w713) -> ("X out"=w748:i32[], "Y out"=w747:i32[], "AnalysisDisplayOutput"=→"AnalysisDisplay":picture)  [unwired: 4 in]
                                n495 = global write "Globaltracker.vi" "index"(w710) -> ()
                                n496 = call "Skipback_171213.vi"("Y out 3"=w747, "X in"=w748, "Skip Back Button"="Skip Back Button", "Boolean in"=w707) -> ("Y out"=w745:i32[], "Y out 2"=w746:i32[])  [unwired: 6 in]
                                n497 = call "Skipforward_171213.vi"("Y out 3"=w745, "Y out 4"=w746, "Skip Forward Button"="Skip Forward Button", "Boolean in"=w706) -> ("Y out"=w743:i32[], "Y out 2"=w744:i32[])  [unwired: 6 in]
                                n498 = call "SeekBack_171213.vi"("Y out 3"=w743, "Y out 4"=w744, "Seek Back Button"="Seek Back Button", "Boolean in"=w705) -> ("Y out"=w740:i32[], "Y out 2"=w742:i32[])  [unwired: 6 in]
                                n499 = control-ref of="Seek Forward Button"() -> (w704:refnum<vi>)
                                n500 = call "SeekForward_171213.vi"("Y in"=w740, "Y out 4"=w742, "Seek Forward Button"="Seek Forward Button", "Boolean in"=w704) -> ("Y out"=w739:i32[], "Y out 3"=w741:i32[])  [unwired: 6 in]
                                n501 = local read "EXIT"() -> (w708:bool)
                                n502 = Wait (ms)(milliseconds to wait=w702) -> ()  [unwired: 1 out]
                                n503 = Or(x=w727, y=w708) -> (x .or. y?=w726:bool)
                                n504 = case shown="False" w726 {
                                frame False {
                                n505 = property on="Start/play" class="Bool (strict)"("Colors [4]"=cluster{u32, u32}[] [{16747264, 16764057}]) -> (error out=w784:errorcluster)  [unwired: 2 in, 1 out]
                                n506 = property on="Stop Button" class="Bool (strict)"("DisabledEnum"=T3."Disabled and Grayed Out" ("Disabled")) -> (error out=w781:errorcluster)  [unwired: 2 in, 1 out]
                                n507 = while {
                                tunnel: [w789] -> w786
                                tunnel: w784 -> [w788]
                                tunnel: w781 -> [w787]
                                tunnel: [w787] -> w779
                                stop <- w791 stop-if-true
                                n508 = local read "Start/play"() -> (w791:bool)
                                n509 = property on="Start/play" class="Bool (strict)"(error in=w788, "Blinking"=TRUE) -> (error out=w789:errorcluster)  [unwired: 1 in, 1 out]
                                }
                                n510 = property on="Start/play" class="Bool (strict)"(error in=w786, "Blinking"=FALSE) -> ()  [unwired: 1 in, 2 out]
                                n511 = property on="Stop Button" class="Bool (strict)"(error in=w779, "DisabledEnum"=T3."Enabled" ("Disabled")) -> ()  [unwired: 1 in, 2 out]
                                }
                                frame True {
                                }
                                }
                                }
                                frame #2 {
                                n512 = call "DisplaySpeedDisplay_171213.vi"("Display Speed"=w792) -> ("PlayBackSpeedDisplay"=→"Playback Speed":string)  [unwired: 10 in]
                                n513 = call "IndexCheckifBelow0_171213.vi"() -> ()  [unwired: 12 in]
                                }
                                frame #3 {
                                n514 = global read "Globaltracker.vi" "index"() -> (w796:i32)
                                n515 = Divide(x=w796, y=80.0) -> (x/y=w798:dbl)
                                n516 = Divide(x=w798, y=60.0) -> (x/y=w800:dbl)
                                n517 = local write "Playback progress (min)"(w800) -> ()
                                }
                              }
                              n518 = local read "EXIT"() -> (w660:bool)
                              n519 = Or(x=w658, y=w660) -> (x .or. y?=w659:bool)
                            }
                          }
                          frame #2 {
                            w803 = 0 ("index")
                            w806 = FALSE
                            n520 = local read "Mousebackground"() -> (w807:picture)
                            n521 = local write "AnalysisDisplay"(w807) -> ()
                            n522 = local write "ProgressBar"(w803) -> ()
                            n523 = local write "Stop Button"(w806) -> ()
                            n524 = local write "Start/play"(w806) -> ()
                            n525 = global write "Globaltracker.vi" "Analysiss"(TRUE ("Anal")) -> ()
                            n526 = global write "Globaltracker.vi" "index"(w803) -> ()
                          }
                          frame #3 {
                            n527 = local read "EXIT"() -> (w810:bool)
                            n528 = case shown="False" w810 {
                              selector: w810 -> [_ w821]
                              tunnel: w808 -> [w812 _]
                              tunnel: [w811 w821] -> w809
                              frame False {
                                n529 = case shown="True" w812 {
                                tunnel: [w813 w817] -> w811
                                frame False {
                                n530 = Two Button Dialog(message="Do you want to load a new recording?", 1:"No" ("F button name (\"Cancel\")"), 2:"Yes" ("T button name (\"OK\")")) -> (T button?=w813:bool)
                                }
                                frame True {
                                n531 = Two Button Dialog(message="Do you want to load a new recording?", 1:"No" ("F button name (\"Cancel\")"), 2:"Yes" ("T button name (\"OK\")")) -> (T button?=w817:bool)
                                }
                                }
                              }
                              frame True {
                              }
                            }
                          }
                        }
                      }
                      "Current Distance\n Traveled (m)" <- w558
                      "Mouse speed (cm/s)" <- w558
                      "Mouse Speed plotted vs time" <- w558
                      "Average Speed (cm/s)" <- w558
                      "Total Distance Traveled (m)" <- w558
                      "Display Speed" <- w558
                      "index" <- w558
                      "date/time" <- "" ("date/time string 2")
                    }
                  }
                  "ProgressBar" <- u16 0 ("ProgressBar")
                }
              }
              n532 = Or(x=w526, y="EXIT") -> (x .or. y?=w524:bool)
            }
          }
        }
      }
    }
    frame #2 {
      n533 = property class="App"() -> ("App.Kind"=w822:T9)  [unwired: 2 in, 2 out]
      n534 = case "Close front panel" shown="\"invalid app kind\", Default" w822 {
        frame "invalid app kind", Default {
          n535 = Open VI Reference(vi path=path "Tracker.vi") -> (vi reference=w824:refnum<vi>)  [unwired: 5 in, 1 out]
          n536 = invoke class="VI" method="FP.Close"(reference=w824) -> ()  [unwired: 2 in, 3 out]
        }
        frame "Development System" {
        }
      }
    }
  }
  n537 = disable-structure shown="Enabled" {
    frame Disabled {
      n538 = Seconds To Date/Time() -> (date time rec=w832:T10)  [unwired: 2 in]
      n539 = Unbundle By Name(w832) -> ("fractional second"=w831:dbl, "second"=w830:i32, "minute"=w829:i32, "hour"=w828:i32)
      n540 = formula code="S=ms+s;\nM=S/60+m;\nH=M/60+h;"("ms"=w831, "s"=w830, "m"=w829, "h"=w828) -> ("M"=w827:dbl, "H"=w826:dbl, "S"=w825:dbl)
      n541 = Bundle("M"=w827, "H"=w826, "S"=w825) -> ()  [unwired: 1 in, 1 out]
    }
    frame Enabled {
    }
  }
